vi "WHD_VEten_0.1.4.WS_BIDIR_Cal_05_03_2020 - modificado.vi"() -> ()   [LabVIEW 2015]
uses:
  <vilib>/LabVIEW Targets/FPGA/cRIO/shared/nicrio_ModuleControls/nicrio_cRIO-9234_DataRatesRing2.ctl
  <vilib>/RTwatchdog.llb/Watchdog expiration actions.ctl
  <vilib>/userdefined/High Color/nirio_resource_hc.ctl
  <vilib>/Platform/TimedLoop/XDataNode/timing_clust.ctl
  <vilib>/Platform/TimedLoop/XDataNode/nitl_modes.ctl
  <vilib>/Platform/TimedLoop/XDataNode/wakeup.ctl
  <vilib>/Analysis/5stat.llb/RMS (DBL).vi
  <vilib>/FPGAPlugInAG/cRIO-9031/niLvFpga_Open_cRIO-9031.vi
  <vilib>/Utility/error.llb/Error Cluster From Error Code.vi
  <vilib>/rvi/errors/niLvFpgaAdjustHostInterfaceError.vi
  <vilib>/FPGAPlugInAG/cRIO-9031/niLvFpga_Run_cRIO-9031.vi
  <vilib>/rvi/interface/common/niFpgaWaitOnOcc.vi
  <vilib>/Utility/file.llb/Write Delimited Spreadsheet (string).vi
  <vilib>/FPGAPlugInAG/cRIO-9031/niLvFpga_Reset_cRIO-9031.vi
  <vilib>/measure/madcrms.llb/Basic Averaged DC-RMS for 1 Chan.vi
  <vilib>/measure/maspectr.llb/FFT Spectrum (Mag-Phase) for 1 Chan.vi
  <vilib>/Utility/config.llb/Write Key (Double).vi
  <vilib>/FPGAPlugInAG/cRIO-9031/niLvFpga_Close_cRIO-9031.vi
  <vilib>/rvi/interface/nirviOpenFPGA/nirviOpenFPGA.xnode
  FPGA Bitfiles/WRDArabia_FPGATarget_FPGA8a2wsBIdirec_pdg683fU6LY.lvbitx
  <vilib>/rvi/interface/nirviReadWriteControl/nirviReadWriteControl.xnode
  <vilib>/rvi/interface/nirviMethod/nirviMethod.xnode
  <vilib>/platform/TimedLoop/XDataNode/XDataNode.xnode
  <vilib>/rvi/interface/nirviCloseFPGA/nirviCloseFPGA.xnode
  <vilib>/rvi/errors/niLvFpgaMergeErrorWithErrorCode.vi
  AURA_Wheel/Json2Labv.lvlib
  AURA_Wheel/AuraWheelAPI/AuraWheel.lvlib
  NiFpgaLv.dll
  <vilib>/FPGAPlugInAG/cRIO-9031/niLvFpga_ConfigureFifo_cRIO-9031.vi
  <vilib>/FPGAPlugInAG/cRIO-9031/niLvFpga_StartFifo_cRIO-9031.vi
  <vilib>/FPGAPlugInAG/cRIO-9031/niLvFpga_ReadFifo_cRIO-9031.vi
  <vilib>/FPGAPlugInAG/cRIO-9031/niLvFpga_StopFifo_cRIO-9031.vi
  <vilib>/measure/NI_MAPro.lvlib
  <vilib>/Analysis/NI_AALPro.lvlib
  <vilib>/Analysis/NI_AALBase.lvlib
  <vilib>/Utility/config.llb/NI_LVConfig.lvlib
  <vilib>/Platform/TimedLoop/XDataNode/XDNodeRunTimeDep.lvlib
  Library/IF2_Reader/IF2_Reader.lvlib
panel:
  out "appended array":string[][](array[string])
  out "TagData out":cluster{"TagCode":string, "FirstSeemUs":u64}[](array[cluster])
  out "error_RFID":errorcluster
  out "Power Status":bool
  out "Diagnostic data":sgl[](array[numeric])
  out "Last Train passes - RFIDs":T1
  out "I2":sgl[](array[numeric])
  out "I1":sgl[](array[numeric])
  out "A8":sgl[](array[numeric])
  out "A7":sgl[](array[numeric])
  out "A6":sgl[](array[numeric])
  out "A5":sgl[](array[numeric])
  out "A4":sgl[](array[numeric])
  out "A3":sgl[](array[numeric])
  out "A2":sgl[](array[numeric])
  out "A1":sgl[](array[numeric])
  out "Accelerometer 8":bool
  out "Accelerometer 7":bool
  out "Accelerometer 6":bool
  out "Accelerometer 5":bool
  out "Accelerometer 4":bool
  out "Accelerometer 3":bool
  out "Accelerometer 2":bool
  out "Accelerometer 1":bool
  out "Wheel detector 2":bool
  out "Wheel Detector 1":bool
  out "Last time checked":string
  out "RFID connection":bool
  out "Internet connection":bool
  out "Inicio diagnosis":timestamp
  out "RFID_status":path=path "c:/RFID/status.csv"
  in  "Diagnosis":bool
  out "T fuera rango":bool
  out "Frequency":dbl[](array[numeric])
  out "Value to compare":dbl[](array[numeric])
  in  "Developer password":string
  out "min":dbl[](array[numeric])
  out "max":dbl[](array[numeric])
  out "median":dbl[](array[numeric])
  out "mean":dbl[](array[numeric])
  in  "Accelerometer":i32=1 min=1 max=8
  out "Low cutoff freq":dbl
  out "noise_range":dbl
  out "Numeric":i32
  out "Calibration parameter":dbl
  out "Accel.detected":i32
  out "Mean\nfrequency":dbl format="%0.2f"
  out "Nº meas":i32
  out "Array":i32[](array[numeric])
  out "sorted array":i32[](array[numeric])
  out "Array 3":i32[](array[numeric])
  out "max value":i32
  out "max index(es)":i32
  out "element":i32
  out "size(s) 3":i32
  out "size(s)":i32[](array[numeric])
  out "Valid\nindex":i32[](array[numeric])
  out "Acquiring time":dbl
  out "Inicio pasada 2":timestamp
  out "calibration log":path
  out "date/time string 2":string
  out "Folder":path
  in  "Developer commad":string
  out "Save calibration":bool
  out "Pattern amplitude (g)":dbl=1.02
  out "Pattern frequency (Hz)":dbl=159.2
  out "Report":string
  out "AURA wheel test":bool
  out "LOG.txt":path
  out "Report_AURA":string
  out "error FPGA":errorcluster
  out "error AURA":errorcluster
  out "error manipulacion archivos":errorcluster
  out "Response headers":string
  out "Max RMS Ruedas":dbl[][](array[numeric])
  out "TAGs LR6":string[](array[string])
  out "TAGs HEX":string[](array[string])
  out "Parar":bool
  out "result":bool
  out "TAGs":string[](array[string])
  out "Temperatura (ºC)":dbl
  out "V (m/s)":dbl
  out "Digital?":bool=TRUE
  out "Watchdog config":T2={"reset"=FALSE, "occurrence"=FALSE, "trigger protocol"=enum."active high", "trigger line"=enum."none", "disable watchdog on VI exit"=TRUE}
  out "Tiempo de adquisicion":dbl=10.0
  out "Adquirir":bool
  out "Nº Ruedas 1":i32
  out "NºRuedas 2":i32
  out "Disco Duro Disponible (bytes)":i64
  out "Buffer Overflow":bool
  out "Buffer Underflow":bool
  out "Archivo\nvalido?":bool
  out "Número de ejes detectados":i32
  out "Ejes_convoy":i32
  out "Tiempo de paso (s)":dbl
  out "created path":path
  out "Nombre de archivo":path[](array[path])
  out "LR6 IP address":string="192.168.106.94"
  out "Port LR6":u16=2001
  out "Frecuencia de muestreo (Hz)":dbl=25600.0
  out "Escaneos de la FIFO por canal":u32=5000
  out "Tiempo extra al detector de paso (s)":dbl=1.0
  out "dt RMS":dbl=256.0
  out "Frecuencia de muestreo y módulo CRIO":T3=2 items=["51.200 kS/s (NI 9234)"=1, "25.600 kS/s (NI 9234)"=2, "17.067 kS/s (NI 9234)"=3, "12.800 kS/s (NI 9234)"=4, "10.240 kS/s (NI 9234)"=5, "8.533 kS/s (NI 9234)"=6, "7.314 kS/s (NI 9234)"=7, "6.400 kS/s (NI 9234)"=8, "5.689 kS/s (NI 9234)"=9, "5.120 kS/s (NI 9234)"=10, "4.654 kS/s (NI 9234)"=11, "4.267 kS/s (NI 9234)"=12, "3.938 kS/s (NI 9234)"=13, "3.657 kS/s (NI 9234)"=14, "3.413 kS/s (NI 9234)"=15, "3.200 kS/s (NI 9234)"=16, "3.012 kS/s (NI 9234)"=17, "2.845 kS/s (NI 9234)"=18, "2.695 kS/s (NI 9234)"=19, "2.560 kS/s (NI 9234)"=20, "2.438 kS/s (NI 9234)"=21, "2.328 kS/s (NI 9234)"=22, "2.226 kS/s (NI 9234)"=23, "2.133 kS/s (NI 9234)"=24, "2.048 kS/s (NI 9234)"=25, "1.969 kS/s (NI 9234)"=26, "1.896 kS/s (NI 9234)"=27, "1.829 kS/s (NI 9234)"=28, "1.765 kS/s (NI 9234)"=29, "1.707 kS/s (NI 9234)"=30, "1.652 kS/s (NI 9234)"=31]
  out "Puerto RFID":u16=2189
  out "IP RFID":string="192.168.106.99"
  out "Offset_rueda WS 2":fxp<+/-,24,-4>=0.004999998956918716 format="%.27g"
  out "Count(mSec)":u32=2
  out "RFID NEM on?":bool
  out "RFID LR6 on?":bool
  out "Canal cero WS1?":bool
  out "Canal cero WS2":bool
  in  "Calibration":bool
  out "Direccion 0?":bool
  out "Boton Adquirir?":bool
  out "RuedaDetectada2?":bool=TRUE
  out "RuedaDetectada1?":bool=TRUE
  out "Timeout ruedas":dbl
  out "Borrar archivos\nadquisicion con error":bool
  out "Able watchdog?":bool
  out "Reset watchdog?":bool
  out "Leer config RFID NEM":bool
  out "bytes to read":i32
  out "DeviceAddress":u8
  out "timeout ms (60000)":i32
  out "Max archivos":u32=2
  out "Bytes libre despues de borrar":u32=2
  out "Bytes min libre":u32=2
  out "Nº de acelerómetros":i32
  out "Nº inductivos":i32
  out "Offset_rueda WS 1":fxp<+/-,24,-4>=0.004999998956918716 format="%.27g"
  out "TAGs_AURAwheel":string[][](array[string])
  out "Plataformas?":bool
  out "Nº Ejes":i32[](array[numeric])
  out "Nº UTs":i32
  out "it-read-LR6":i32[](array[numeric])
  out "it-LR6":i32
  out "RFID_LR6_Error":errorcluster
  out "Series_flota":string[](array[string])
  out "Tabla_flota":string[][](array[string])
  out "Puntos medios de las ventanas":dbl[][](array[numeric])
  out "configuration file path":path=path "c:/Parametros.cfg"
  out "IP synchr":string
  out "data":cluster{"status":string}
  out "confRFID":path=path "c:/RFID/TAGS.csv"
  out "TAGS leidos":path=path "c:/RFID/TAGS.csv"
  out "Use Aura?":bool
  out "Parametros AuraWheel":string[](array[string])
  out "Parámetros acelerómetros":dbl[](array[numeric])
  out "Fin":bool
  out "Contador":i32=1
  out "Path LOG":path=path "c:/TEST"
  out "Fallo fotocelula":bool
  out "Path_Borrar":path=path "c:/Trenes"
  out "Longitud de la unidad":dbl
  out "Aviso no detección":string
  out "Time to Acquire Block (ms)":i32
  out "Distancia de acelerómetros":dbl[](array[numeric])
  out "Block Size":u32
  out "Distancias generales":dbl[](array[numeric])
  out "Reset del controlador":bool
  out "Parar la aplicación":bool
  out "date/time string":string
  out "Timeout ruedas":bool
  out "Tiempo":dbl
  out "Inicio pasada":timestamp
  out "Ultimo TEST":timestamp
  out "DC OK":string
  out "Aviso temperatura":string
  out "connection ID":refnum<k5>
  # "Date"
  # "Train"
  # "TAG1"
  # "TAG2"
  # "To check the status of the UPS please check the following LEDs physically in the system:"
  # "10. Bar graph showing the current available supply of the UPS (each bar is a 20%)"
  # "12. Red LED: alarm"
  # "13. Yellow LED: battery working mode"
  # "16. Green LED: Power In OK, mains mode"
  # "Calibration - Noise analysis"
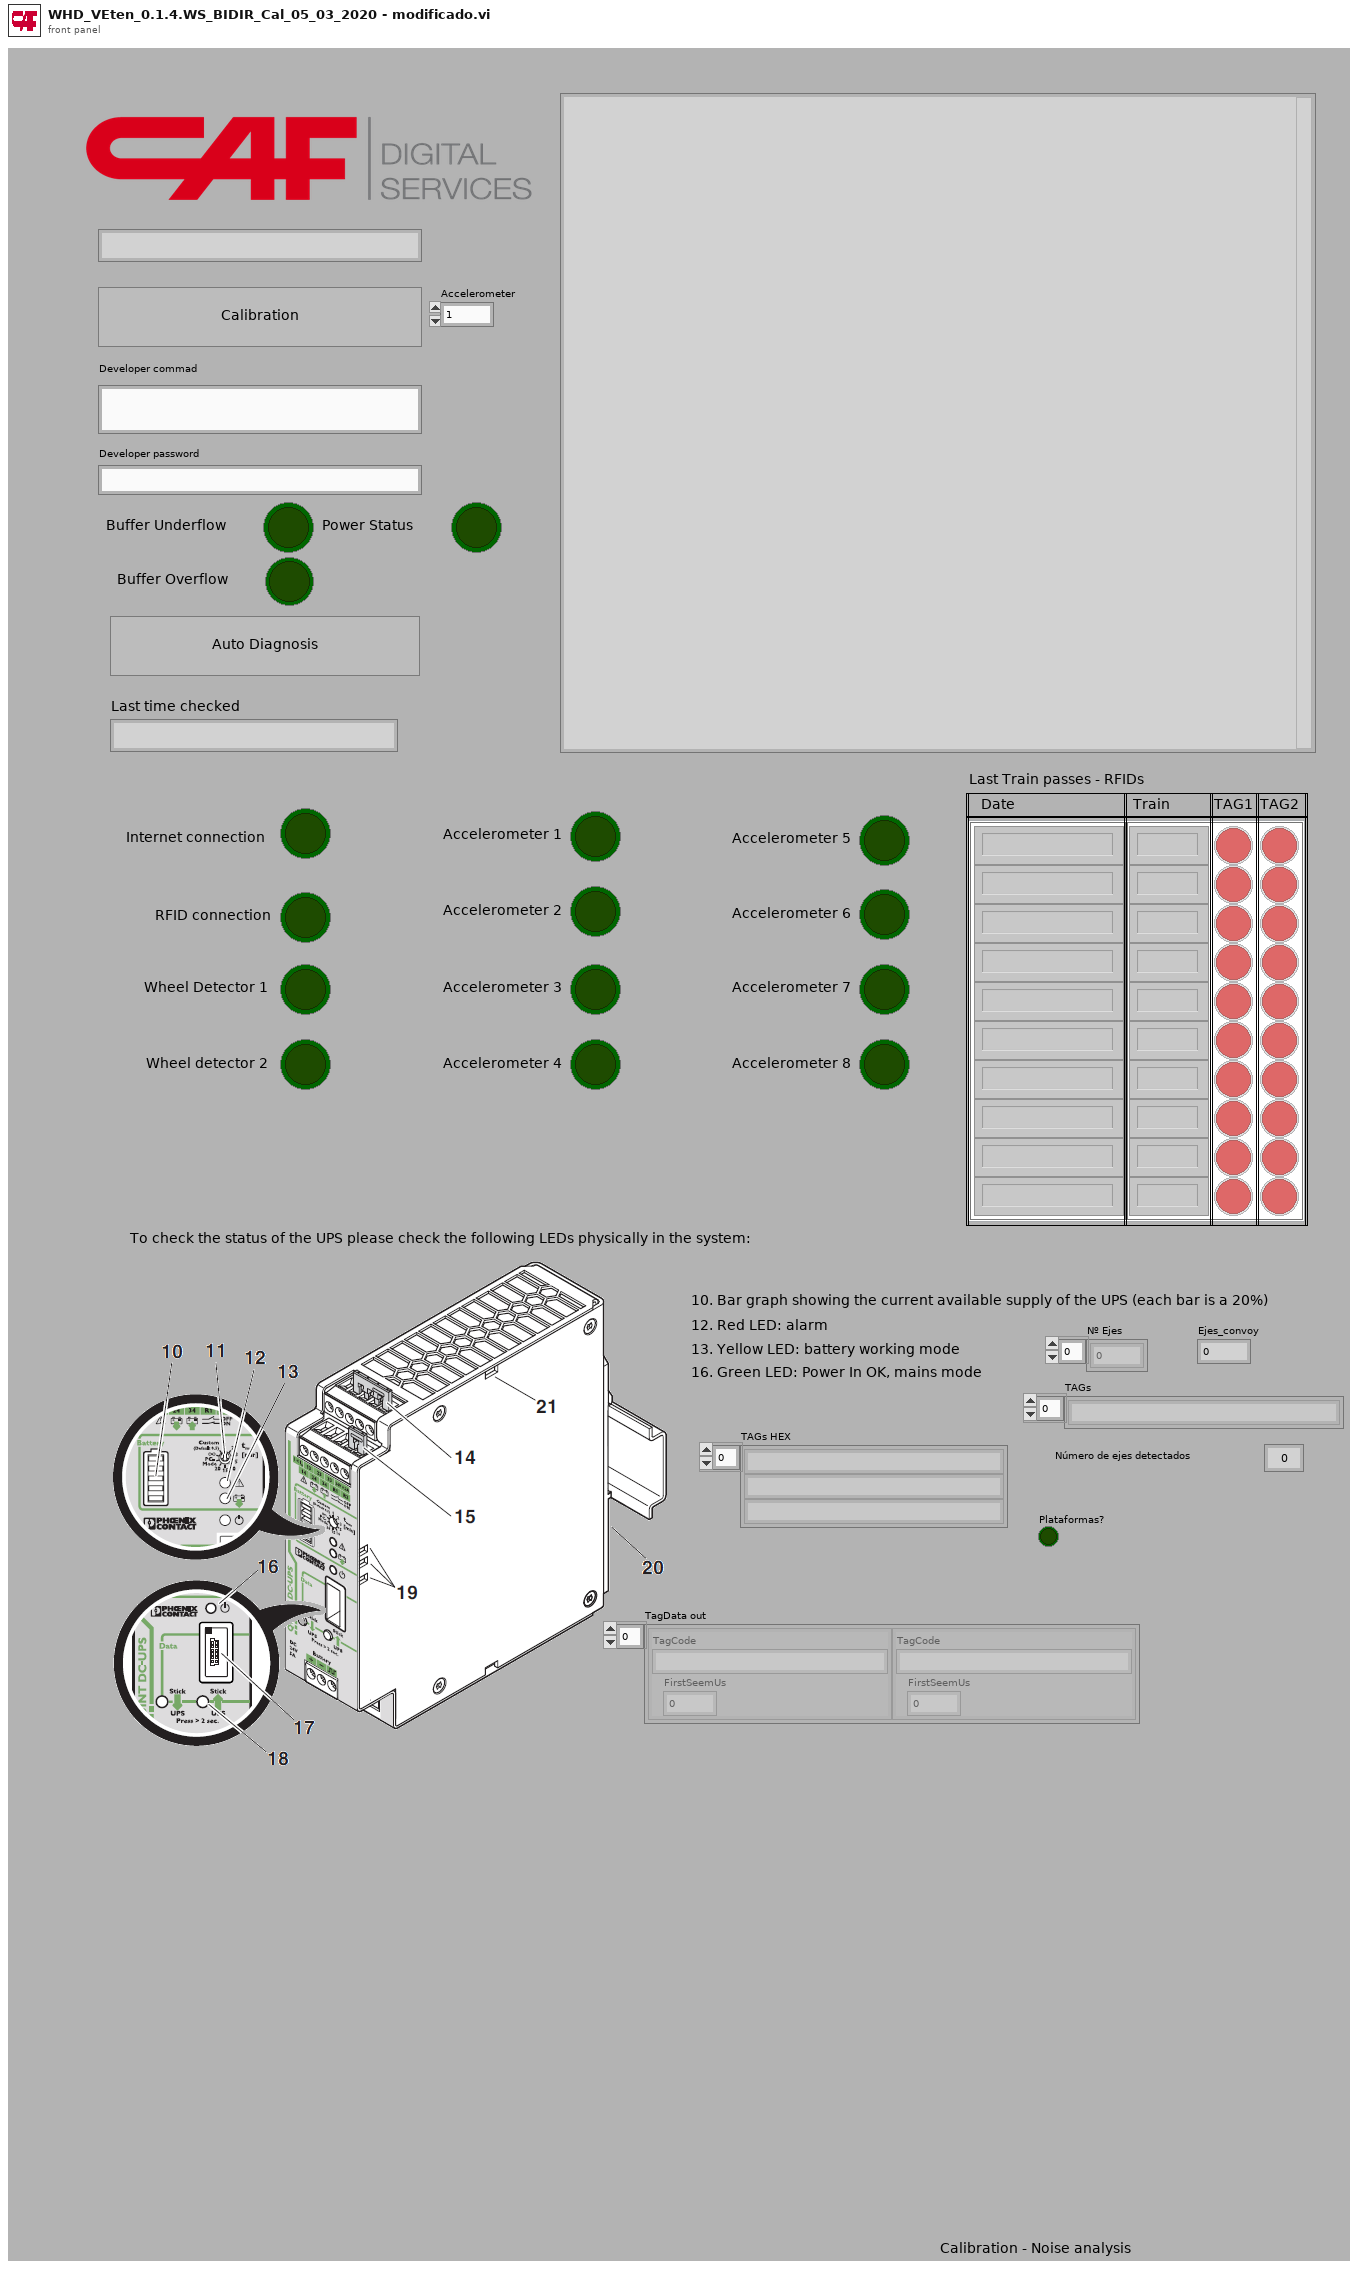
[diagram p1: front panel]
types:
  T1 = cluster{"Array 3":bool[], "Array 4":string[], "Array 6":string[], "Array 5":bool[]}
  T2 = typedef "Watchdog expiration actions.ctl" = cluster{"reset":bool, "occurrence":bool, "trigger protocol":enum16{"active high", "active low", "open collector"}, "trigger line":enum16{"none", "line 0", "line 1", "line 2", "line 3", "line 4", "line 5", "line 6", "line 7", "SMB line 0"}, "disable watchdog on VI exit":bool}
  T3 = typedef "nicrio_cRIO-9234_DataRatesRing2.ctl" = u8
  T4 = typedef "nirio_resource_hc.ctl" = tag
  T5 = enum16{"open", "replace", "create", "open or create", "replace or create", "replace or create with confirmation"}
  T6 = enum16{"big-endian, network order", "native, host order", "little-endian"}
  T7 = typedef "XDNodeRunTimeDep.lvlib/timing_clust.ctl" = cluster{"Expected End [f-1]":u64, "Actual End [f-1]":u64, "Finished Late? [f-1]":bool, "Expected End [i-1]":u64, "Actual End [i-1]":u64, "Finished Late? [i-1]":bool, "Expected Start [i]":u64, "Actual Start [i]":u64, "Expected Start [f]":u64, "Actual Start [f]":u64, "Source Name":string, "Structure Name":string, "Period":i64, "Deadline":i64, "Offset":i64, "Start":i64, "Priority":i32, "Timeout":i32, "Mode":T8, "Wakeup Reason":T9, "Error":errorcluster, "Source Type":string, "Secondary Source Type":string, "Global End Time":u64, "Global Start Time":u64, "Frame Duration":u64, "Iteration Duration":u64, "Assigned CPU":i32, "I/O Scan Engine Mode":u32}
  T8 = typedef "XDNodeRunTimeDep.lvlib/nitl_modes.ctl" = enum32{"No Change", "Process missed periods, maintain original phase", "Discard missed periods, maintain original phase", "Process missed periods, ignore original phase", "Discard missed periods, ignore original phase"}
  T9 = typedef "XDNodeRunTimeDep.lvlib/wakeup.ctl" = enum32{"Normal", "Aborted", "Asynchronous wakeup", "Timing source error", "Timed loop error", "Timeout"}
  T10 = cluster{"error IO":errorcluster, bool[], u32[], string[], dbl[]}
  T11 = cluster{"error out":errorcluster, dbl[], "Normalized Tags":string[], "Direccion 0?":bool}
  T12 = cluster{"g_ts":dbl, "p_sp":dbl, "p_tp":dbl, "p_tg":cluster{"tg_n":dbl, "tg_t":string}[], "p_ax":cluster{"ax_n":dbl, "ax_sp":dbl, "ax_wh":cluster{"wh_p":dbl, "wh_a1":dbl, "wh_a2":dbl, "wh_a3":dbl, "wh_a4":dbl}[]}[]}
  T13 = typedef "NI_LVConfig.lvlib/Config Data RefNum.ctl" = refnum<k1>
  T14 = cluster{"IP":string, "Port":u16, "ReaderConfigFile":path, "ROspecConfigFile":path}
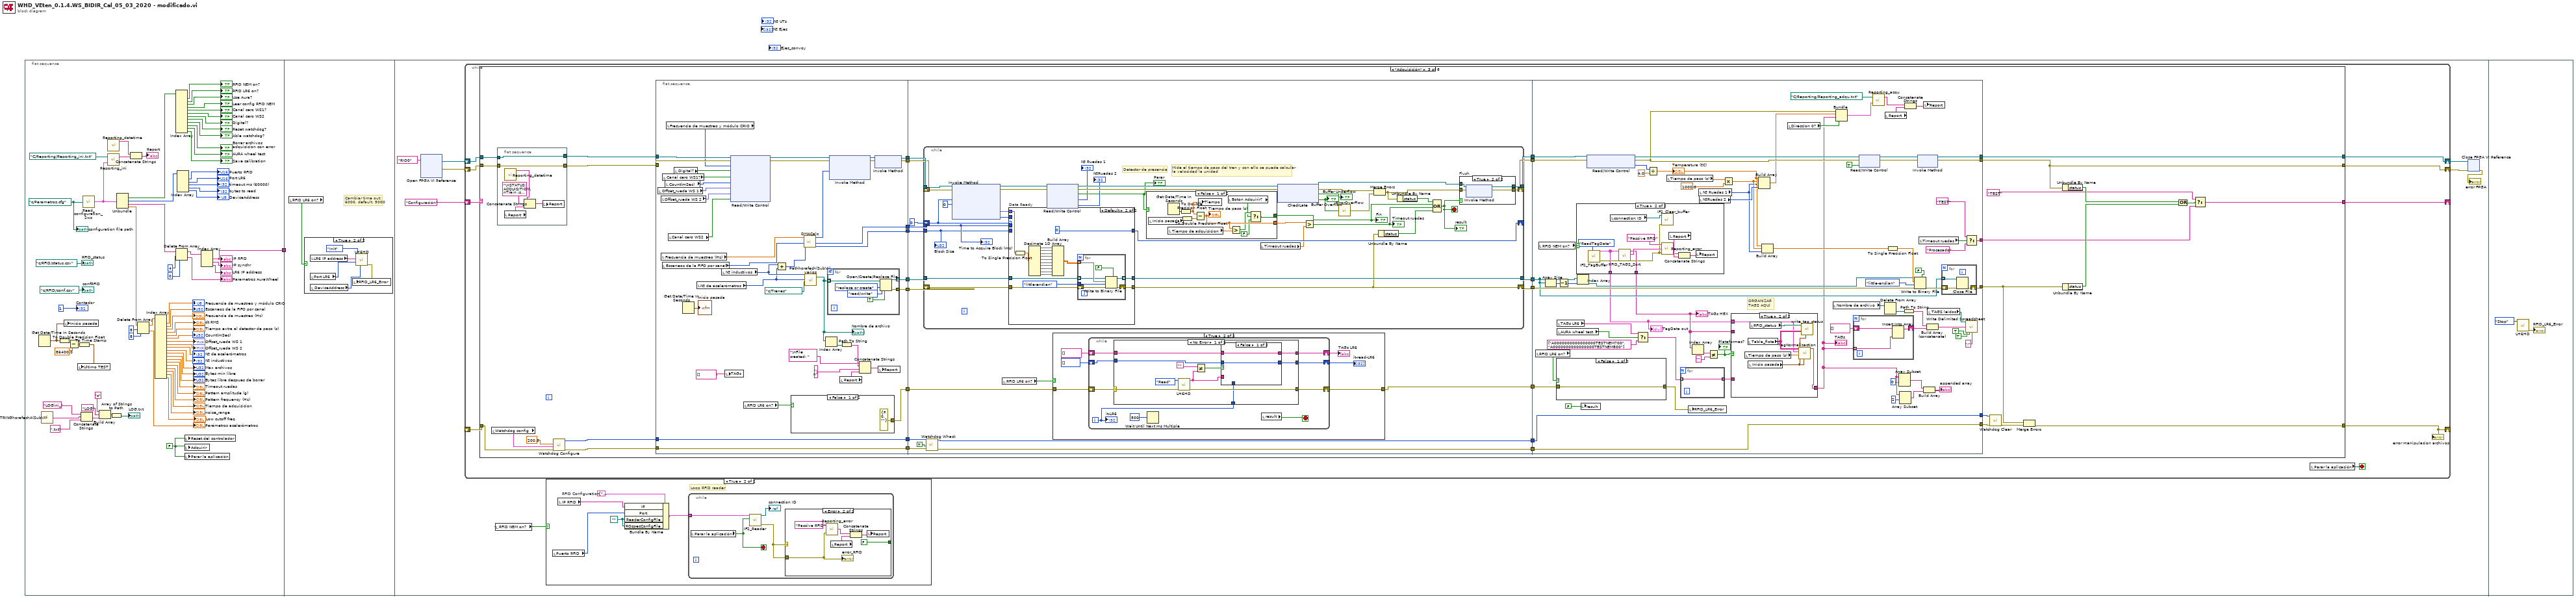
[diagram p0: block diagram]
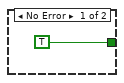
[diagram p4: hidden frame]
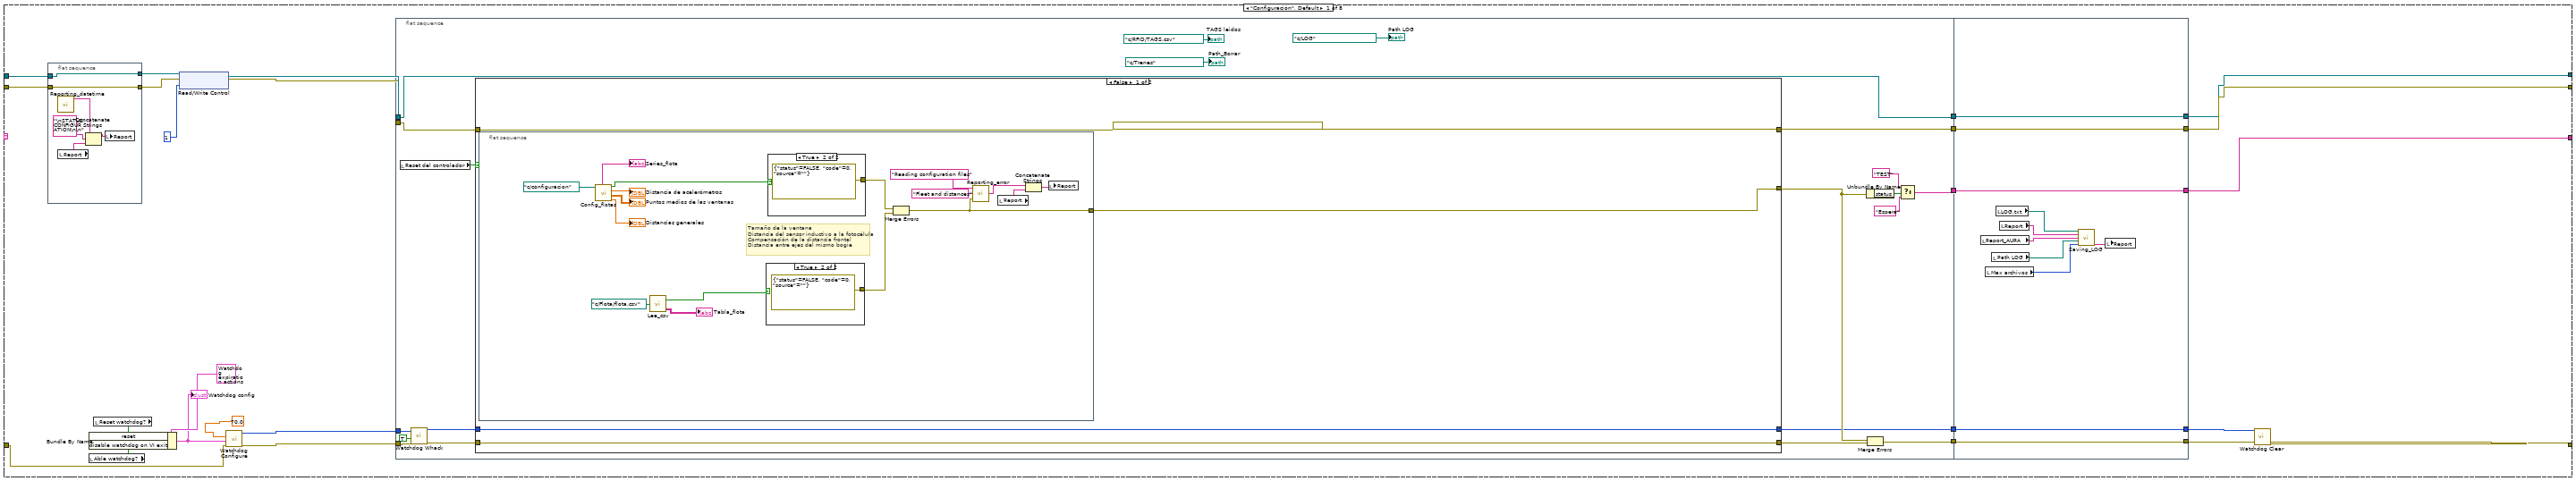
[diagram p5: hidden frame]
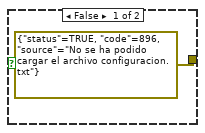
[diagram p6: hidden frame]
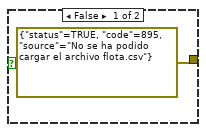
[diagram p7: hidden frame]
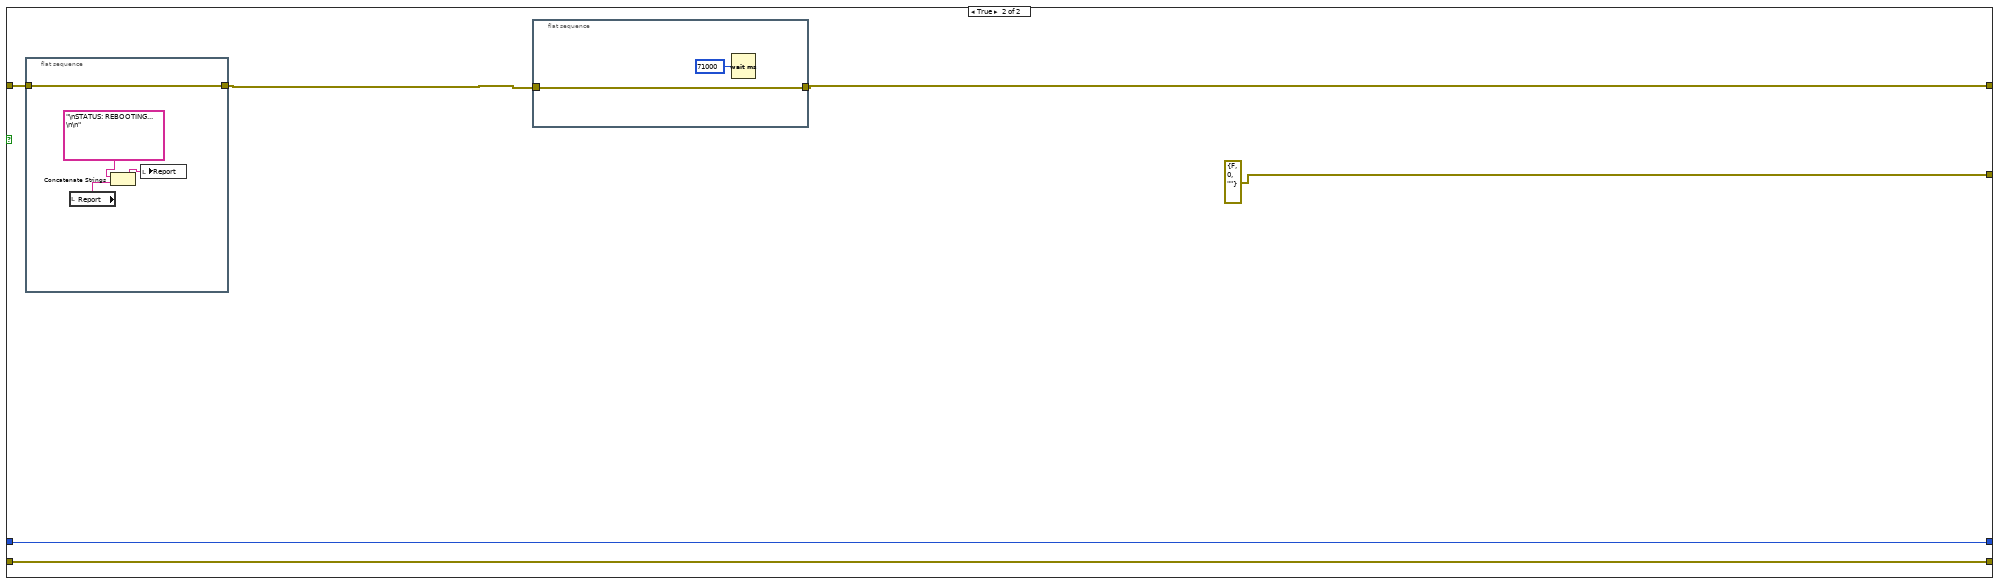
[diagram p8: hidden frame]
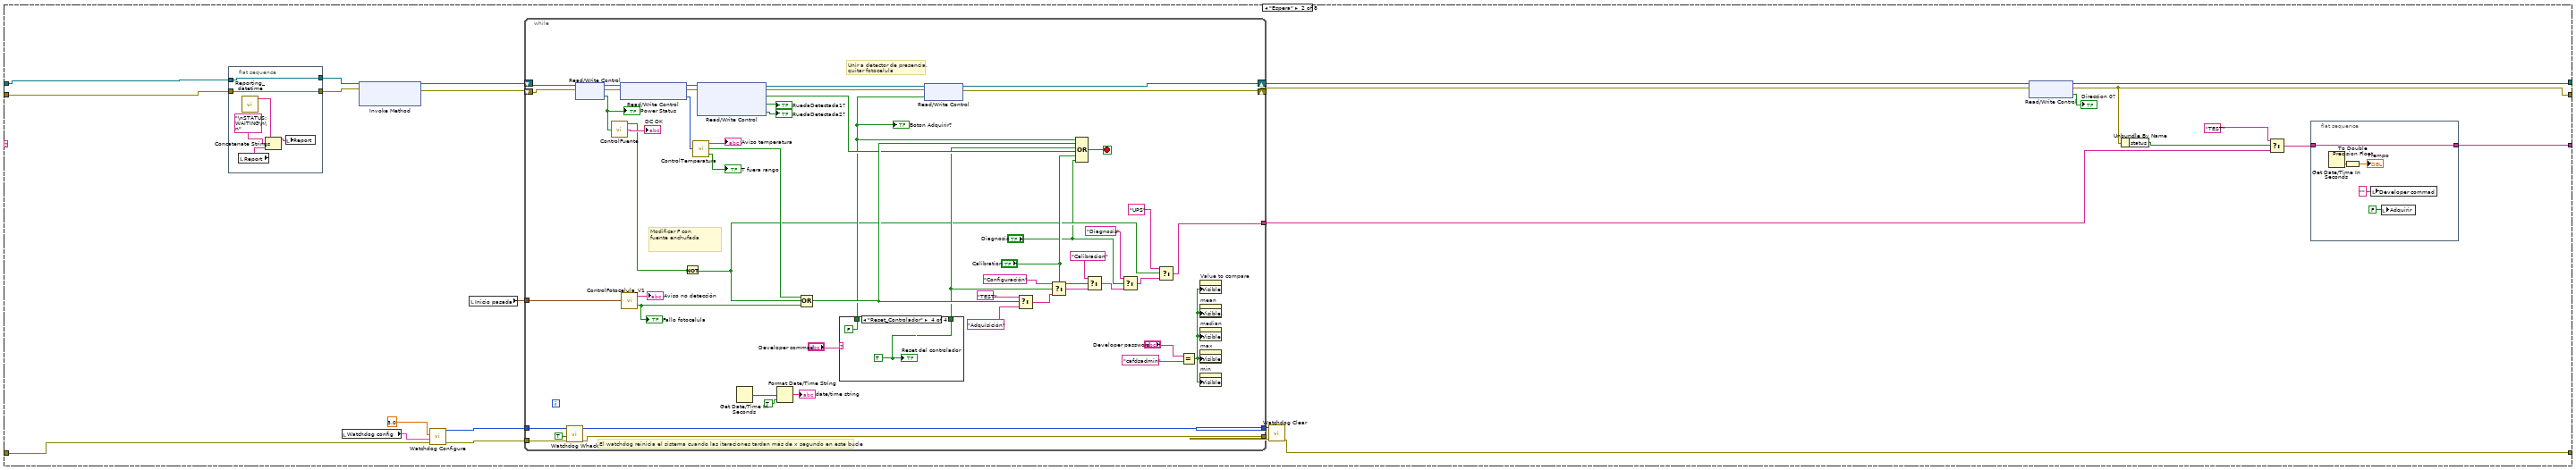
[diagram p9: hidden frame]
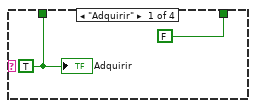
[diagram p10: hidden frame]
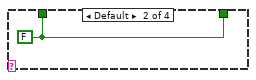
[diagram p11: hidden frame]
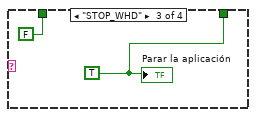
[diagram p12: hidden frame]
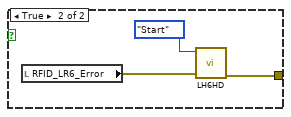
[diagram p13: hidden frame]
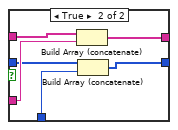
[diagram p15: hidden frame]
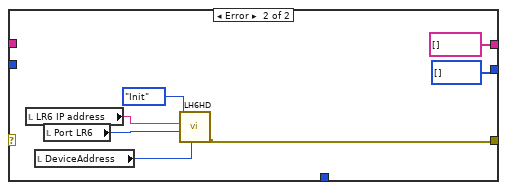
[diagram p16: hidden frame]
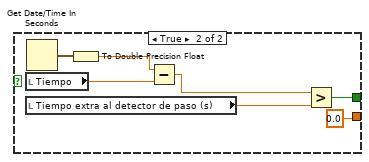
[diagram p17: hidden frame]
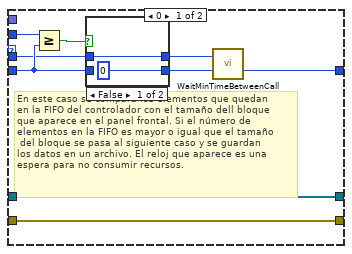
[diagram p18: hidden frame]
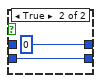
[diagram p19: hidden frame]
diagram:
  n1 = flat-sequence {
    tunnel: [w5] -> w1
    tunnel: w1 -> [_]
    frame #0 {
      w6 = FALSE ("Reset del controlador")
      w67 = path "c:/Parametros.cfg" ("configuration file path")
      n2 = Get Date/Time In Seconds() -> (seconds since 1Jan1904=w72:timestamp)
      n3 = call "STRINGhorafechA(SubVI).vi"() -> ("STRINGhora_fecha"=w17:string)
      n4 = To Double Precision Float(number=w72) -> (double precision float=w74:dbl)
      n5 = local write "Inicio pasada"(w72) -> ()
      n6 = Subtract(x=w74, y=86400.0) -> (x-y=w73:dbl)
      n7 = To Time Stamp(1:w73) -> (0:w71:timestamp)
      n8 = local write "Ultimo TEST"(w71) -> ()
      n9 = Concatenate Strings("LOGini_" ("string"), w17, ".txt" ("string")) -> (w19:string)
      n10 = call "Read_configuration_2ws.vi"("configuration file path"=w67) -> ("output cluster"=w23:T10)
      n11 = Build Array("c", "LOG" ("element"), w19) -> (w16:string[])
      n12 = call "Reporting_ini.vi"("Configuration cluster"=w23, "address repoting"=path "C:/Reporting/Reporting_ini.txt" ("file (use dialog)")) -> ("Reporting"=w22:string)  [unwired: 1 in]
      n13 = call "Reporting_datetime.vi"() -> ("String"=w20:string)  [unwired: 11 in]
      n14 = Array of Strings to Path(0:w16) -> (2:→"LOG.txt":path)  [unwired: 1 out]
      n15 = Unbundle(w23) -> (w70:bool[], w69:u32[], w62:string[], w66:dbl[])  [unwired: 1 out]
      n16 = Concatenate Strings(w20, w22) -> (→"Report":string)
      n17 = Delete From Array(array=w66, length=8, index=8) -> (deleted portion=→"Parámetros acelerómetros":dbl[], array with subset deleted=w65:dbl[])
      n18 = Index Array(array=w65) -> (element #1=→"Frecuencia de muestreo y módulo CRIO":dbl, element #2=→"Escaneos de la FIFO por canal":dbl, element #3=→"Frecuencia de muestreo (Hz)":dbl, element #4=→"dt RMS":dbl, element #5=→"Tiempo extra al detector de paso (s)":dbl, element #6=→"Count(mSec)":dbl, element #7=→"Offset_rueda WS 1":dbl, element #8=→"Offset_rueda WS 2":dbl, element #9=→"Nº de acelerómetros":dbl, element #10=→"Nº inductivos":dbl, element #11=→"Max archivos":dbl, element #12=→"Bytes min libre":dbl, element #13=→"Bytes libre despues de borrar":dbl, element #14=→"Timeout ruedas":dbl, element #15=→"Pattern amplitude (g)":dbl, element #16=→"Pattern frequency (Hz)":dbl, element #17=→"Tiempo de adquisicion":dbl, element #18=→"noise_range":dbl, element #19=→"Low cutoff freq":dbl)  [unwired: 19 in]
      n19 = Index Array(array=w70) -> (element #1=→"RFID NEM on?":bool, element #2=→"RFID LR6 on?":bool, element #3=→"Use Aura?":bool, element #4=→"Leer config RFID NEM":bool, element #5=→"Canal cero WS1?":bool, element #6=→"Canal cero WS2":bool, element #7=→"Digital?":bool, element #8=→"Reset watchdog?":bool, element #9=→"Able watchdog?":bool, element #10=→"Borrar archivos\nadquisicion con error":bool, element #11=→"AURA wheel test":bool, element #12=→"Save calibration":bool)  [unwired: 12 in]
      n20 = Delete From Array(array=w62, length=4, index=0) -> (deleted portion=→"Parametros AuraWheel":string[], array with subset deleted=w61:string[])
      n21 = Index Array(array=w69) -> (element #1=→"Puerto RFID":u32, element #2=→"Port LR6":u32, element #3=→"timeout ms (60000)":u32, element #4=→"bytes to read":u32, element #5=→"DeviceAddress":u32)  [unwired: 5 in]
      n22 = local write "Reset del controlador"(w6) -> ()
      n23 = local write "Adquirir"(w6) -> ()
      n24 = local write "Parar la aplicación"(w6) -> ()
      n25 = Index Array(array=w61) -> (element #1=w5:string, element #2=→"IP synchr":string, element #3=→"LR6 IP address":string)  [unwired: 3 in]
      "IP RFID" <- w5
      "Contador" <- 1
      "confRFID" <- path "c:/RFID/conf.csv" ("file path (use dialog)")
      "configuration file path" <- w67
      "RFID_status" <- path "c:/RFID/status.csv" ("file path (use dialog)")
    }
    frame #1 {
      # "Cambiar time out:\n6000, default, 5000"
      n26 = local read "RFID LR6 on?"() -> (w76:bool)
      n27 = case shown="True" w76 {
        frame False {
        }
        frame True {
          n28 = local read "LR6 IP address"() -> (w77:string)
          n29 = local read "Port LR6"() -> (w78:u16)
          n30 = local read "DeviceAddress"() -> (w79:u8)
          n31 = call "LH6HD.vi"("DeviceAddress"=w79, "Reader Port"=w78, "IP Address"=w77, "Action"=enum16{"Init", "Start", "Read", "Stop", "Exit"}."Init") -> ("error out"=w81:errorcluster)  [unwired: 6 in, 1 out]
          n32 = local write "RFID_LR6_Error"(w81) -> ()
        }
      }
    }
    frame #2 {
      n33 = xnode "Open FPGA VI Reference"("resource name"=T4 "RIO0") -> ("FPGA VI Reference Out"=w89:refnum<k20>, "error out"=w88:errorcluster)  [unwired: 1 in]
      n34 = while {
        shift-right: [w107] -> _
        shift-left: "Configuración" -> [w114]
        shift-right: [w106] -> w85
        shift-left: w89 -> [w113]
        shift-right: [w108] -> w84
        shift-left: w88 -> [w112]
        shift-right: [w111] -> _
        shift-left: _ -> [w110]
        stop <- w109 stop-if-true
        n35 = case shown="\"Adquisición\"" w114 {
          tunnel: [w129 w232 w328 w682 w931 "Espera" "Espera" ("t") "Espera" ("t")] -> w107
          tunnel: [w139 w221 w342 w671 w930 w999 w1795 w1818] -> w106
          tunnel: [w140 w220 w343 w669 w929 w997 w1794 w1827] -> w108
          tunnel: w113 -> [w123 w219 w314 w672 w930 w1009 w1796 w1836]
          tunnel: w112 -> [w122 w218 w313 w670 w922 w1008 w1791 w1838]
          tunnel: [w136 w226 w340 w667 w921 w998 w1792 w1819] -> w111
          tunnel: w110 -> [w128 w231 w324 w681 w918 w998 w1792 w1819]
          frame "Configuración", Default {
            n36 = flat-sequence {
              tunnel: w123 -> [w146]
              tunnel: w122 -> [w145]
              tunnel: [w146] -> w121
              tunnel: [w145] -> w120
              frame #0 {
                n37 = call "Reporting_datetime.vi"() -> ("String"=w141:string)  [unwired: 11 in]
                n38 = local read "Report"() -> (w142:string)
                n39 = Concatenate Strings(w141, "\nSTATUS: CONFIGURATION\n\n", w142) -> (w144:string)
                n40 = local write "Report"(w144) -> ()
              }
            }
            n41 = local read "Able watchdog?"() -> (w133:bool)
            n42 = local read "Reset watchdog?"() -> (w134:bool)
            n43 = Bundle By Name(cluster=T2 {"reset"=FALSE, "occurrence"=FALSE, "trigger protocol"=enum."active high", "trigger line"=enum."none", "disable watchdog on VI exit"=TRUE} ("expiration actions"), "reset"=w134, "disable watchdog on VI exit"=w133) -> (w127:T2)
            "Watchdog config" <- w127
            n44 = xnode "Read/Write Control"("FPGA VI Reference In"=w121, "error in"=w120, "Cycles to Filter"=u16 1) -> ("FPGA VI Reference Out"=w132:refnum<k20>, "error out"=w131:errorcluster)
            n45 = call <vilib>:"Watchdog Configure.vi"("error in (no error)"=w128, "expiration actions"=w127, "timeout (1 sec)"=70.0) -> ("error out"=w124:errorcluster, "watchdogID"=w125:u64)  [unwired: 1 in, 2 out]
            n46 = flat-sequence {
              tunnel: w132 -> [w158]
              tunnel: w131 -> [w155]
              tunnel: w125 -> [w148]
              tunnel: w124 -> [w147]
              tunnel: [w157] -> w119
              tunnel: [w165] -> w118
              tunnel: [w158] -> w117
              tunnel: [w160] -> w116
              tunnel: [w152] -> w115
              tunnel: [w210] -> w138
              tunnel: [w211] -> w137
              tunnel: [w212] -> w139
              tunnel: [w213] -> w129
              tunnel: [w214] -> w140
              tunnel: w119 -> [w214]
              tunnel: w118 -> [w213]
              tunnel: w117 -> [w212]
              tunnel: w116 -> [w211]
              tunnel: w115 -> [w210]
              frame #0 {
                n47 = local read "Reset del controlador"() -> (w154:bool)
                n48 = call <vilib>:"Watchdog Whack.vi"("error in (no error)"=w147, "reset watchdog after expire? (F)"=TRUE, "watchdogID in"=w148) -> ("error out"=w150:errorcluster, "watchdogID out"=w151:u64)  [unwired: 2 in, 1 out]
                n49 = case shown="False" w154 {
                  tunnel: w155 -> [w170 w193]
                  tunnel: [w170 w196] -> w157
                  tunnel: [w167 errorcluster {"status"=FALSE, "code"=0, "source"=""} ("error IO")] -> w156
                  tunnel: [w169 w195] -> w152
                  tunnel: w151 -> [w169 w195]
                  tunnel: w150 -> [w168 w194]
                  tunnel: [w168 w194] -> w149
                  frame False {
                    n50 = flat-sequence {
                      tunnel: [w171] -> w167
                      frame #0 {
                        # "Tamaño de la ventana\nDistancia del sensor inductivo a la fotocélula\nCompensación de la distancia frontal\nDistancia entre ejes del mismo bogie"
                        n51 = call "Config_flotas.vi"("file path (dialog if empty)"=path "c:/configuracion") -> ("Distancias generales"=→"Distancias generales":dbl[], "Puntos medios de las ventanas"=→"Puntos medios de las ventanas":dbl[][], "Distancia de acelerómetros"=→"Distancia de acelerómetros":dbl[], "Distacias y medidas de dispositivos"=w184:bool, "Series_flota"=→"Series_flota":string[])  [unwired: 3 in]
                        n52 = call "Lee_csv.vi"("Path"=path "c:/Flota/flota.csv") -> ("Tabla_flota"=→"Tabla_flota":string[][], "Lectura_OK?"=w181:bool)
                        n53 = case shown="True" w181 {
                          tunnel: [errorcluster {"status"=TRUE, "code"=895, "source"="No se ha podido cargar el archivo flota.csv"} ("error out") errorcluster {"status"=FALSE, "code"=0, "source"=""} ("error out")] -> w185
                          frame False {
                          }
                          frame True {
                          }
                        }
                        n54 = case shown="True" w184 {
                          tunnel: [errorcluster {"status"=TRUE, "code"=896, "source"="No se ha podido cargar el archivo configuracion.txt"} ("error out") errorcluster {"status"=FALSE, "code"=0, "source"=""} ("error out")] -> w186
                          frame False {
                          }
                          frame True {
                          }
                        }
                        n55 = Merge Errors(w186, w185) -> (w171:errorcluster)
                        n56 = call "Reporting_error.vi"("error out 2"=w171, "Concept explanation"="Fleet and distances", "Concept"="Reading configuration files") -> ("Reporting"=w173:string)
                        n57 = local read "Report"() -> (w172:string)
                        n58 = Concatenate Strings(w173, w172) -> (w174:string)
                        n59 = local write "Report"(w174) -> ()
                      }
                    }
                  }
                  frame True {
                    n60 = flat-sequence {
                      tunnel: w193 -> [w201]
                      tunnel: [w201] -> w192
                      frame #0 {
                        n61 = local read "Report"() -> (w200:string)
                        n62 = Concatenate Strings("\nSTATUS: REBOOTING...\n\n", w200) -> (w198:string)
                        n63 = local write "Report"(w198) -> ()
                      }
                    }
                    n64 = flat-sequence {
                      tunnel: [w203] -> w196
                      tunnel: w192 -> [w203]
                      frame #0 {
                        n65 = Wait (ms)(milliseconds to wait=u32 71000) -> ()  [unwired: 1 out]
                      }
                    }
                  }
                }
                n66 = Unbundle By Name(w156) -> ("status"=w166:bool)
                n67 = Merge Errors(w156, w149) -> (w160:errorcluster)
                n68 = Select(t="TEST", s=w166, f="Espera") -> (s? t:f=w165:string)
                "Path_Borrar" <- path "c:/Trenes" ("file path (use dialog)")
                "Path LOG" <- path "c:/LOG" ("file path (use dialog)")
                "TAGS leidos" <- path "c:/RFID/TAGS.csv" ("file path (use dialog)")
              }
              frame #1 {
                n69 = local read "Report_AURA"() -> (w207:string)
                n70 = local read "Max archivos"() -> (w208:u32)
                n71 = local read "Path LOG"() -> (w209:path)
                n72 = local read "LOG.txt"() -> (w204:path)
                n73 = local read "Report"() -> (w206:string)
                n74 = call "Saving_LOG.vi"("Path"=w204, "Report"=w206, "Report AURA"=w207, "Path Carpeta"=w209, "Nº Archivos Max"=w208) -> ("Report"=w205:string)  [unwired: 9 in, 1 out]
                n75 = local write "Report"(w205) -> ()
              }
            }
            n76 = call <vilib>:"Watchdog Clear.vi"("error in (no error)"=w137, "watchdogID in"=w138) -> ("error out"=w136:errorcluster)  [unwired: 5 in]
          }
          frame "Espera" {
            n77 = flat-sequence {
              tunnel: w219 -> [w245]
              tunnel: w218 -> [w244]
              tunnel: [w245] -> w217
              tunnel: [w244] -> w216
              frame #0 {
                n78 = local read "Report"() -> (w241:string)
                n79 = call "Reporting_datetime.vi"() -> ("String"=w240:string)  [unwired: 11 in]
                n80 = Concatenate Strings(w240, "\nSTATUS: WAITING\n\n", w241) -> (w243:string)
                n81 = local write "Report"(w243) -> ()
              }
            }
            n82 = local read "Watchdog config"() -> (w225:T2)
            n83 = xnode "Invoke Method"("FPGA VI Reference In"=w217, "error in"=w216) -> ("FPGA VI Reference Out"=w235:refnum<k20>, "error out"=w234:errorcluster)  [unwired: 1 in]
            n84 = call <vilib>:"Watchdog Configure.vi"("error in (no error)"=w231, "expiration actions"=w225, "timeout (1 sec)"=3.0) -> ("error out"=w230:errorcluster, "watchdogID"=w229:u64)  [unwired: 1 in, 2 out]
            n85 = local read "Inicio pasada"() -> (w239:timestamp)
            n86 = while {
              tunnel: [w261] -> w238
              shift-right: [w276] -> w222
              shift-left: w235 -> [w284]
              shift-right: [w275] -> w215
              shift-left: w234 -> [w283]
              tunnel: w239 -> [w287]
              tunnel: w230 -> [w273]
              tunnel: w229 -> [w274]
              tunnel: [w272] -> w228
              tunnel: [w271] -> w227
              stop <- w266 stop-if-true
              # "Modificar F con\nfuente enchufada"
              # "Unir a detector de presencia,\nquitar fotocelula"
              # "El watchdog reinicia el sistema cuando las iteraciones tardan más de x segundo en este bucle"
              n87 = call <vilib>:"Watchdog Whack.vi"("error in (no error)"=w273, "reset watchdog after expire? (F)"=TRUE, "watchdogID in"=w274) -> ("error out"=w271:errorcluster, "watchdogID out"=w272:u64)  [unwired: 2 in, 1 out]
              n88 = xnode "Read/Write Control"("FPGA VI Reference In"=w284, "error in"=w283) -> ("FPGA VI Reference Out"=w296:refnum<k20>, "error out"=w295:errorcluster, "DC OK"=w251:bool)
              "Power Status" <- w251
              n89 = call "ControlFuente.vi"("DC OK 3"=w251) -> ("DC OK 2"=w262:bool, "DC OK"=→"DC OK":string)  [unwired: 1 out]
              n90 = xnode "Read/Write Control"("FPGA VI Reference In"=w296, "error in"=w295) -> ("FPGA VI Reference Out"=w291:refnum<k20>, "error out"=w290:errorcluster, "Chassis Temperature"=w298:i16)
              n91 = call "ControlFotocelula_V1.vi"("Tiempo de entrada a espera"=w287) -> ("Aviso no detección"=→"Aviso no detección":string, "Boolean"=w288:bool)
              "Fallo fotocelula" <- w288
              n92 = Not(x=w262) -> (.not. x?=w260:bool)
              n93 = call "ControlTemperatura.vi"("Chassis Temperature"=w298) -> ("Aviso temperatura"=→"Aviso temperatura":string, "Boolean"=w292:bool, "T fuera rango"=→"T fuera rango":bool)
              n94 = xnode "Read/Write Control"("FPGA VI Reference In"=w291, "error in"=w290) -> ("FPGA VI Reference Out"=w286:refnum<k20>, "error out"=w285:errorcluster, "Detector de presencia"=w279:bool, "RuedaDetectada1?"=→"RuedaDetectada1?":bool, "RuedaDetectada2?"=→"RuedaDetectada2?":bool)
              n95 = Get Date/Time In Seconds() -> (seconds since 1Jan1904=w281:timestamp)
              n96 = Format Date/Time String(seconds (now)=w281, UTC format=TRUE) -> (date/time string=→"date/time string":string)  [unwired: 1 in]
              n97 = Compound Arithmetic op=OR(w292, w260, w288) -> (w289:bool)
              n98 = case shown="\"Reset_Controlador\"" "Developer commad" {
                tunnel: [w305 w306 FALSE ("Adquirir") FALSE ("Adquirir")] -> w265
                tunnel: [FALSE ("Adquirir") w306 w307 w309] -> w264
                frame "Adquirir" {
                  w305 = TRUE ("Adquirir")
                  "Adquirir" <- w305
                }
                frame Default {
                  w306 = FALSE ("Adquirir")
                }
                frame "STOP_WHD" {
                  w307 = TRUE ("Adquirir")
                  "Parar la aplicación" <- w307
                }
                frame "Reset_Controlador" {
                  w309 = TRUE ("Adquirir")
                  "Reset del controlador" <- w309
                }
              }
              "Boton Adquirir?" <- w265
              n99 = xnode "Read/Write Control"("FPGA VI Reference In"=w286, "error in"=w285, "Fotocélula"=w265) -> ("FPGA VI Reference Out"=w276:refnum<k20>, "error out"=w275:errorcluster)
              n100 = Select(t="TEST", s=w289, f="Adquisición") -> (s? t:f=w300:string)
              n101 = Select(t="Configuración", s=w264, f=w300) -> (s? t:f=w269:string)
              n102 = Compound Arithmetic op=OR(w265, w289, w264, w279, "Calibration", "Diagnosis") -> (w266:bool)
              n103 = Select(t="Calibracion", s="Calibration", f=w269) -> (s? t:f=w255:string)
              n104 = Select(t="Diagnosis", s="Diagnosis", f=w255) -> (s? t:f=w253:string)
              n105 = Select(t="UPS", s=w260, f=w253) -> (s? t:f=w261:string)
              n106 = Equal?(x="Developer password", y="cafdsadmin") -> (x = y?=w257:bool)
              n107 = property on="Value to compare" class="Arr (strict)"("Visible"=w257) -> ()  [unwired: 2 in, 2 out]
              n108 = property on="mean" class="Arr (strict)"("Visible"=w257) -> ()  [unwired: 2 in, 2 out]
              n109 = property on="median" class="Arr (strict)"("Visible"=w257) -> ()  [unwired: 2 in, 2 out]
              n110 = property on="max" class="Arr (strict)"("Visible"=w257) -> ()  [unwired: 2 in, 2 out]
              n111 = property on="min" class="Arr (strict)"("Visible"=w257) -> ()  [unwired: 2 in, 2 out]
            }
            n112 = call <vilib>:"Watchdog Clear.vi"("error in (no error)"=w227, "watchdogID in"=w228) -> ("error out"=w226:errorcluster)  [unwired: 5 in]
            n113 = xnode "Read/Write Control"("FPGA VI Reference In"=w222, "error in"=w215) -> ("FPGA VI Reference Out"=w221:refnum<k20>, "error out"=w220:errorcluster, "Direccion 0?"=→"Direccion 0?":bool)
            n114 = Unbundle By Name(w220) -> ("status"=w237:bool)
            n115 = Select(t="TEST", s=w237, f=w238) -> (s? t:f=w233:string)
            n116 = flat-sequence {
              tunnel: [w249] -> w232
              tunnel: w233 -> [w249]
              frame #0 {
                n117 = Get Date/Time In Seconds() -> (seconds since 1Jan1904=w250:timestamp)
                n118 = To Double Precision Float(number=w250) -> (double precision float=→"Tiempo":dbl)
                n119 = local write "Developer commad"("" ("Developer commad")) -> ()
                n120 = local write "Adquirir"(FALSE ("Adquirir")) -> ()
              }
            }
          }
          frame "Adquisición" {
            n121 = local read "Watchdog config"() -> (w325:T2)
            n122 = flat-sequence {
              tunnel: w314 -> [w354]
              tunnel: w313 -> [w353]
              tunnel: [w354] -> w312
              tunnel: [w353] -> w311
              frame #0 {
                n123 = local read "Report"() -> (w350:string)
                n124 = call "Reporting_datetime.vi"() -> ("String"=w349:string)  [unwired: 11 in]
                n125 = Concatenate Strings(w349, "\nSTATUS: ACQUISITION\nTrain is passing\n\n", w350) -> (w352:string)
                n126 = local write "Report"(w352) -> ()
              }
            }
            n127 = call <vilib>:"Watchdog Configure.vi"("error in (no error)"=w324, "expiration actions"=w325, "timeout (1 sec)"=200.0) -> ("error out"=w322:errorcluster, "watchdogID"=w323:u64)  [unwired: 1 in, 2 out]
            n128 = flat-sequence {
              tunnel: w311 -> [w389]
              tunnel: w312 -> [w390]
              tunnel: [w388] -> w339
              tunnel: [w387] -> w338
              tunnel: [w386] -> w337
              tunnel: [w385] -> w336
              tunnel: [w384] -> w335
              tunnel: [w383] -> w334
              tunnel: [w373] -> w327
              tunnel: w323 -> [w372]
              tunnel: w322 -> [w371]
              tunnel: [w372] -> w321
              tunnel: [w371] -> w320
              tunnel: [w405] -> w348
              tunnel: [w422] -> w347
              tunnel: [w421] -> w346
              tunnel: [w420] -> w345
              tunnel: [w413] -> w344
              tunnel: w339 -> [w419]
              tunnel: w338 -> [w418]
              tunnel: w337 -> [w417]
              tunnel: w336 -> [w416]
              tunnel: w335 -> [w415]
              tunnel: w334 -> [w414]
              tunnel: w327 -> [w411]
              tunnel: [w410] -> w326
              tunnel: w321 -> [w409]
              tunnel: w320 -> [w408]
              tunnel: [w406] -> w319
              tunnel: w348 -> [w591]
              tunnel: w347 -> [w588]
              tunnel: w346 -> [w587]
              tunnel: w345 -> [w603]
              tunnel: [w625] -> w331
              tunnel: w344 -> [w627]
              tunnel: [w618] -> w341
              tunnel: [w619] -> w343
              tunnel: [w620] -> w342
              tunnel: w326 -> [w599]
              tunnel: w319 -> [w592]
              tunnel: [w592] -> w317
              tunnel: [w591] -> w316
              frame #0 {
                n129 = local read "Offset_rueda WS 1"() -> (w366:fxp<+/-,24,-4>)
                n130 = local read "Offset_rueda WS 2"() -> (w367:fxp<+/-,24,-4>)
                n131 = local read "Frecuencia de muestreo (Hz)"() -> (w381:dbl)
                n132 = local read "Escaneos de la FIFO por canal"() -> (w370:u32)
                n133 = local read "Canal cero WS1?"() -> (w375:bool)
                n134 = local read "Count(mSec)"() -> (w374:u32)
                n135 = local read "Frecuencia de muestreo y módulo CRIO"() -> (w377:T3)
                n136 = local read "Canal cero WS2"() -> (w365:bool)
                n137 = local read "Digital?"() -> (w376:bool)
                n138 = Get Date/Time In Seconds() -> (seconds since 1Jan1904=→"Inicio pasada":timestamp)
                n139 = local read "Nº de acelerómetros"() -> (w363:i32)
                n140 = local read "Nº inductivos"() -> (w364:i32)
                n141 = local write "TAGs"(string[] [] ("TAGs")) -> ()
                n142 = xnode "Read/Write Control"("FPGA VI Reference In"=w390, "error in"=w389, "Data Rate"=w377, "Digital?"=w376, "Canal cero WS1?"=w375, "Count(mSec)"=w374, "Offset_WS1"=w366, "Offset_WS2"=w367, "Canal cero WS2?"=w365) -> ("FPGA VI Reference Out"=w380:refnum<k20>, "error out"=w379:errorcluster)
                n143 = local read "RFID LR6 on?"() -> (w368:bool)
                n144 = Add(x=w364, y=w363) -> (x+y=w369:i32)
                n145 = case shown="False" w368 {
                  tunnel: [errorcluster {"status"=FALSE, "code"=0, "source"=""} ("error out") w395] -> w373
                  frame False {
                  }
                  frame True {
                    n146 = local read "RFID_LR6_Error"() -> (w396:errorcluster)
                    n147 = call "LH6HD.vi"("error in (no error)"=w396, "Action"=enum16{"Init", "Start", "Read", "Stop", "Exit"}."Start") -> ("error out"=w395:errorcluster)  [unwired: 8 in, 1 out]
                  }
                }
                n148 = call "DMACalc.vi"("Number of Channels"=w369, "Number of Samples"=w370, "Rate (Hz)"=w381) -> ("Block Size"=w385:u32, "Time to Acquire Block (ms)"=w386:i32, "Host Buffer Size"=w391:u32)  [unwired: 6 in]
                n149 = call "Pathhorafech(SubVI)_varios.vi"("Folder path"=path "c:/Trenes", "Nº de acelerómetros"=w363, "Nº inductivos"=w364) -> ("Acel_Paths"=w359:path[])  [unwired: 1 in, 1 out]
                "Nombre de archivo" <- w359
                n150 = Index Array(array=w359) -> (element=w358:path)  [unwired: 1 in]
                n151 = for {
                  tunnel: w359 -> [w400] mode=indexing
                  tunnel: [w399] -> w384 mode=indexing
                  tunnel: [w398] -> w383
                  n152 = Open/Create/Replace File(file path (use dialog)=w400, operation (0:open)=T5."replace or create", access (0:read/write)=enum16{"read/write", "read-only", "write-only"}."read/write", disable buffering (F)=TRUE) -> (refnum out=w399:refnum<file>, error out=w398:errorcluster)  [unwired: 1 in, 2 out]
                }
                n153 = xnode "Invoke Method"("FPGA VI Reference In"=w380, "error in"=w379, "Requested Depth"=w391) -> ("FPGA VI Reference Out"=w393:refnum<k20>, "error out"=w392:errorcluster)  [unwired: 1 out]
                n154 = local read "Report"() -> (w362:string)
                n155 = Path To String(path=w358) -> (string=w356:string)
                n156 = Concatenate Strings("\nFile created: ", w356, "\n", w362) -> (w361:string)
                n157 = xnode "Invoke Method"("FPGA VI Reference In"=w393, "error in"=w392) -> ("FPGA VI Reference Out"=w388:refnum<k20>, "error out"=w387:errorcluster)
                n158 = local write "Report"(w361) -> ()
              }
              frame #1 {
                n159 = while "Data Acquisition" {
                  tunnel: w419 -> [w473]
                  shift-right: [w497] -> _
                  shift-left: u32 0 ("t") -> [w493]
                  tunnel: w417 -> [w498]
                  tunnel: w416 -> [w496]
                  shift-right: [w499] -> w421
                  shift-left: w418 -> [w490]
                  tunnel: [w494] -> w422
                  tunnel: w415 -> [w477]
                  tunnel: [w478] -> w420
                  shift-right: [w476] -> w413
                  shift-left: w414 -> [w486]
                  stop <- w495 stop-if-true
                  # "Detector de presencia"
                  # "Mide el tiempo de paso del tren y con ello se puede calcular\nla velocidad la unidad"
                  n160 = xnode "Invoke Method"("FPGA VI Reference In"=w473, "error in"=w490, "Number of Elements"=w493, "Timeout (ms)"=0) -> ("FPGA VI Reference Out"=w470:refnum<k20>, "error out"=w475:errorcluster, "Data"=w489:fxp<+/-,24,4>[], "Elements Remaining"=w491:u32)
                  n161 = case "Data Ready" shown="Default" w493 {
                    tunnel: w498 -> [w521 _]
                    tunnel: [w520 u32 0 ("t")] -> w497
                    tunnel: w496 -> [w522 _]
                    tunnel: w491 -> [w519 _]
                    tunnel: w489 -> [_ w544]
                    tunnel: w486 -> [w518 w543]
                    tunnel: [w518 w545] -> w476
                    tunnel: w477 -> [w517 w542]
                    tunnel: [w517 w541] -> w478
                    frame 0 {
                      # "En este caso se compara los elementos que quedan\nen la FIFO del controlador con el tamaño dell bloque\nque aparece en el panel frontal. Si el número de \nelementos en la FIFO es mayor o igual que el tamaño\n del bloque se pasa al siguiente caso y se guardan \nlos datos en un archivo. El reloj que aparece es una\nespera para no consumir recursos."
                      n162 = Greater Or Equal?(x=w519, y=w522) -> (x >= y?=w523:bool)
                      n163 = case shown="False" w523 {
                        tunnel: [u32 0 ("Block Size") w527] -> w520
                        tunnel: [w526 0 ("t")] -> w524
                        tunnel: w521 -> [w526 _]
                        tunnel: w522 -> [_ w527]
                        frame False {
                        }
                        frame True {
                        }
                      }
                      n164 = call "WaitMinTimeBetweenCall.vi"("Minimum ms between calls"=w524) -> ()  [unwired: 2 in]
                    }
                    frame Default {
                      n165 = To Single Precision Float(number=w544) -> (single precision float=w531:sgl[])
                      n166 = Decimate 1D Array(w531) -> (w537:sgl[], w540:sgl[], w539:sgl[], w538:sgl[], w536:sgl[], w535:sgl[], w534:sgl[], w533:sgl[], w532:sgl[], w529:sgl[])
                      n167 = Build Array(w537, w540, w539, w538, w536, w535, w534, w533, w532, w529) -> (w530:sgl[][])
                      n168 = for {
                        tunnel: T6."little-endian" ("byte order (0:big-endian, network order)") -> [w554]
                        shift-right: [w548] -> w545
                        shift-left: w543 -> [w549]
                        tunnel: w530 -> [w552] mode=indexing
                        tunnel: w542 -> [w551] mode=indexing
                        tunnel: [w550] -> w541 mode=indexing
                        n169 = Write to Binary File(file (use dialog)=w551, data=w552, error in=w549, 5:FALSE ("prepend array or string size? (T)"), 9:w554) -> (refnum out=w550:refnum<file>, error out=w548:errorcluster)  [unwired: 2 out]
                      }
                    }
                  }
                  n170 = xnode "Read/Write Control"("FPGA VI Reference In"=w470, "error in"=w475) -> ("FPGA VI Reference Out"=w488:refnum<k20>, "error out"=w487:errorcluster, "Parar"=w466:bool, "Nº Ruedas 1"=→"Nº Ruedas 1":i32, "NºRuedas 2"=→"NºRuedas 2":i32)
                  "Parar" <- w466
                  n171 = case shown="False" w466 {
                    tunnel: [w504 w512] -> w467
                    tunnel: [w505 0.0] -> w481
                    frame False {
                      n172 = local read "Inicio pasada"() -> (w508:timestamp)
                      n173 = Get Date/Time In Seconds() -> (seconds since 1Jan1904=w507:timestamp)
                      n174 = local read "Tiempo de adquisicion"() -> (w500:dbl)
                      n175 = To Double Precision Float(number=w507) -> (double precision float=w506:dbl)
                      n176 = To Double Precision Float(number=w508) -> (double precision float=w509:dbl)
                      n177 = Subtract(x=w506, y=w509) -> (x-y=w505:dbl)
                      "Tiempo de paso (s)" <- w505
                      n178 = local write "Tiempo"(w506) -> ()
                      n179 = local read "Boton Adquirir?"() -> (w501:bool)
                      n180 = Greater?(x=w505, y=w500) -> (0:w503:bool)
                      n181 = Select(t=w503, s=w501, f=FALSE) -> (s? t:f=w504:bool)
                    }
                    frame True {
                      n182 = local read "Tiempo"() -> (w516:dbl)
                      n183 = local read "Tiempo extra al detector de paso (s)"() -> (w511:dbl)
                      n184 = Get Date/Time In Seconds() -> (seconds since 1Jan1904=w513:timestamp)
                      n185 = To Double Precision Float(number=w513) -> (double precision float=w514:dbl)
                      n186 = Subtract(x=w514, y=w516) -> (x-y=w515:dbl)
                      n187 = Greater?(x=w515, y=w511) -> (0:w512:bool)
                    }
                  }
                  "Fin" <- w467
                  n188 = local read "Timeout ruedas"() -> (w465:dbl)
                  n189 = xnode ("CheckLate")("FPGA VI Reference In"=w488, "error in"=w487) -> ("FPGA VI Reference Out"=w472:refnum<k20>, "error out"=w483:errorcluster, "Buffer Underflow"=→"Buffer Underflow":bool, "Buffer Overflow"=w474:bool)
                  "Buffer Overflow" <- w474
                  n190 = Greater?(x=w481, y=w465) -> (0:w479:bool)
                  "Timeout ruedas" <- w479
                  n191 = call "ErrorOverFlow.vi"("Buffer Overflow"=w474) -> ("error out"=w482:errorcluster)
                  n192 = Merge Errors(w483, w482) -> (w471:errorcluster)
                  n193 = Unbundle By Name(w476) -> ("status"=w480:bool)
                  n194 = Unbundle By Name(w471) -> ("status"=w485:bool)
                  n195 = Compound Arithmetic op=OR(w485, w467, w479, w480) -> (w495:bool)
                  "result" <- w495
                  n196 = case "Flush" shown="True" w495 {
                    tunnel: [w555 w560] -> w499
                    tunnel: [w556 w559] -> w494
                    tunnel: w472 -> [w556 w558]
                    tunnel: w471 -> [w555 w557]
                    frame False {
                    }
                    frame True {
                      n197 = xnode "Invoke Method"("FPGA VI Reference In"=w558, "error in"=w557) -> ("FPGA VI Reference Out"=w559:refnum<k20>, "error out"=w560:errorcluster)
                    }
                  }
                  "Block Size" <- w496
                  "Time to Acquire Block (ms)" <- w498
                }
                n198 = call <vilib>:"Watchdog Whack.vi"("error in (no error)"=w408, "reset watchdog after expire? (F)"=TRUE, "watchdogID in"=w409) -> ("error out"=w405:errorcluster, "watchdogID out"=w406:u64)  [unwired: 2 in, 1 out]
                n199 = local read "RFID LR6 on?"() -> (w404:bool)
                n200 = case shown="True" w404 {
                  tunnel: w411 -> [w423 w429]
                  tunnel: [w423 w428] -> w410
                  frame False {
                  }
                  frame True {
                    n201 = while {
                      shift-right: [w436] -> w428
                      shift-left: w429 -> [w437]
                      shift-right: [w435] -> w426
                      shift-left: string[] [] -> [w434]
                      shift-right: [w430] -> w424
                      shift-left: i32[] [] -> [w431]
                      i -> [w432]
                      stop <- w433 stop-if-true
                      n202 = case shown="No Error" w437 {
                        selector: w437 -> [w448 _]
                        tunnel: [w447 w463] -> w436
                        tunnel: [w443 string[] []] -> w435
                        tunnel: w434 -> [w442 _]
                        tunnel: w432 -> [w441 _]
                        tunnel: w431 -> [w440 _]
                        tunnel: [w439 i32[] []] -> w430
                        frame No Error {
                          n203 = call "LH6HD.vi"("error in (no error)"=w448, "Action"=enum16{"Init", "Start", "Read", "Stop", "Exit"}."Read") -> ("error out"=w447:errorcluster, "Tag"=w444:string)  [unwired: 8 in]
                          n204 = Not Equal?(x="", y=w444) -> (x != y?=w445:bool)
                          n205 = case shown="False" w445 {
                            tunnel: w444 -> [_ w457]
                            tunnel: [w451 w456] -> w443
                            tunnel: w442 -> [w451 w455]
                            tunnel: w441 -> [_ w452]
                            tunnel: w440 -> [w450 w454]
                            tunnel: [w450 w453] -> w439
                            frame False {
                            }
                            frame True {
                              n206 = Build Array (concatenate)(w455, w457) -> (w456:string[])
                              n207 = Build Array (concatenate)(w454, w452) -> (w453:i32[])
                            }
                          }
                        }
                        frame Error {
                          n208 = local read "LR6 IP address"() -> (w460:string)
                          n209 = local read "DeviceAddress"() -> (w458:u8)
                          n210 = local read "Port LR6"() -> (w461:u16)
                          n211 = call "LH6HD.vi"("DeviceAddress"=w458, "Reader Port"=w461, "IP Address"=w460, "Action"=enum16{"Init", "Start", "Read", "Stop", "Exit"}."Init") -> ("error out"=w463:errorcluster)  [unwired: 6 in, 1 out]
                        }
                      }
                      n212 = Wait Until Next ms Multiple(millisecond multiple=u32 500) -> ()  [unwired: 1 out]
                      n213 = local read "result"() -> (w433:bool)
                      "it-LR6" <- w432
                    }
                    "TAGs LR6" <- w426
                    "it-read-LR6" <- w424
                  }
                }
              }
              frame #2 {
                # "ORGANIZAR\nTAGS AQUÍ"
                n214 = local read "RFID LR6 on?"() -> (w589:bool)
                n215 = local read "RFID NEM on?"() -> (w590:bool)
                n216 = Array Size(array=w603) -> (size(s)=w601:i32)
                n217 = case shown="False" w589 {
                  tunnel: w599 -> [w633 w639]
                  tunnel: [w633 w634] -> w598
                  frame False {
                  }
                  frame True {
                    n218 = call "LH6HD.vi"("error in (no error)"=w639, "Action"=enum16{"Init", "Start", "Read", "Stop", "Exit"}."Stop") -> ("error out"=w634:errorcluster)  [unwired: 8 in, 1 out]
                    n219 = call "Reporting_error.vi"("error out 2"=w634, "Concept"="Active RFID") -> ("Reporting"=w636:string)  [unwired: 1 in]
                    n220 = local read "Report"() -> (w637:string)
                    n221 = Concatenate Strings(w636, w637) -> (w635:string)
                    n222 = local write "Report"(w635) -> ()
                  }
                }
                n223 = local read "TAGs LR6"() -> (w569:string[])
                n224 = local read "AURA wheel test"() -> (w568:bool)
                n225 = Decrement(x=w601) -> (x-1=w602:i32)
                n226 = case shown="True" w590 {
                  tunnel: [string[] [] ("TagArray") w646] -> w572
                  tunnel: [cluster{"TagCode":string, "FirstSeemUs":u64}[] [] ("TagData out") w645] -> w571
                  frame False {
                  }
                  frame True {
                    n227 = call "IF2_TagBuffer.vi"("Action"=enum16{"Init", "WriteTagData", "ReadTagData"}."ReadTagData") -> ("error out"=w644:errorcluster, "TagData out"=w645:cluster{"TagCode":string, "FirstSeemUs":u64}[])  [unwired: 9 in]
                    n228 = local read "connection ID"() -> (w643:refnum<k5>)
                    n229 = call "RFID_TAGS_Sort.vi"("TagData in"=w645) -> ("TagString"=w647:string, "TagArray"=w646:string[])  [unwired: 9 in]
                    n230 = call "IF2_Clear_buffer.vi"("error in (no error)"=w644, "TCP Network Connection in"=w643) -> ()  [unwired: 8 in, 2 out]
                    n231 = call "Reporting_error.vi"("error out 2"=w644, "Concept explanation"=w647, "Concept"="Passive RFID") -> ("Reporting"=w650:string)
                    n232 = local read "Report"() -> (w651:string)
                    n233 = Concatenate Strings(w650, w651) -> (w649:string)
                    n234 = local write "Report"(w649) -> ()
                  }
                }
                "TAGs HEX" <- w572
                "TagData out" <- w571
                n235 = Index Array(array=w603, index=w602) -> (element=w611:refnum<file>)
                n236 = local write "result"(FALSE ("result")) -> ()
                n237 = xnode "Read/Write Control"("FPGA VI Reference In"=w588, "error in"=w587) -> ("FPGA VI Reference Out"=w624:refnum<k20>, "error out"=w585:errorcluster, "Chassis Temperature"=w632:i16)
                n238 = Select(t=w569, s=w568, f=string[] ["A0000000000000000TESTNEM700", "A0000000000000000TESTNEM800"]) -> (s? t:f=w573:string[])
                n239 = Divide(x=w632, y=4.0) -> (x/y=w582:dbl)
                "Temperatura (ºC)" <- w582
                n240 = local read "Tiempo de paso (s)"() -> (w622:dbl)
                n241 = for {
                  tunnel: w573 -> [w653] mode=indexing
                  tunnel: [w653] -> w561 mode=indexing
                }
                n242 = local write "RFID_LR6_Error"(w598) -> ()
                n243 = Index Array(array=w572) -> (element=w597:string)  [unwired: 1 in]
                n244 = local read "Nº Ruedas 1"() -> (w580:i32)
                n245 = local read "NºRuedas 2"() -> (w583:i32)
                n246 = Not Equal?(x=w597, y="" ("delimiter (\\t)")) -> (x != y?=w595:bool)
                "Plataformas?" <- w595
                n247 = Multiply(x=w622, y=1000.0) -> (x*y=w581:dbl)
                n248 = case shown="True" w595 {
                  tunnel: w561 -> [w654 _]
                  tunnel: [w654 w655] -> w565
                  tunnel: w571 -> [_ w656]
                  tunnel: w572 -> [_ _]
                  frame False {
                  }
                  frame True {
                    n249 = local read "Tiempo de paso (s)"() -> (w660:dbl)
                    n250 = local read "Tabla_flota"() -> (w658:string[][])
                    n251 = local read "Inicio pasada"() -> (w659:timestamp)
                    n252 = local read "RFID_status"() -> (w657:path)
                    n253 = call "TagNormalizaction.vi"("Inicio pasada"=w659, "Tiempo de paso (s)"=w660, "TagData in"=w656, "Tabla_flota"=w658) -> ("Normalized Tags"=w655:string[])  [unwired: 5 in, 2 out]
                    n254 = call "write_tag_status.vi"("Inicio pasada"=w659, "Tabla_flota"=w658, "file path (use dialog)"=w657) -> ()  [unwired: 8 in]
                  }
                }
                "TAGs" <- w565
                n255 = Build Array(w582, w581, w580, w583) -> (w584:dbl[])
                n256 = Build Array(w582, w581, w580) -> (w579:dbl[])
                n257 = local read "Direccion 0?"() -> (w578:bool)
                n258 = local read "Nombre de archivo"() -> (w610:path[])
                n259 = Bundle("error out"=w585, w584, "Normalized Tags"=w565, "Direccion 0?"=w578) -> (w577:T11)  [unwired: 1 in]
                n260 = for {
                  shift-right: [w666] -> w616
                  shift-left: string[] [] -> [w665]
                  tunnel: w565 -> [w664] mode=indexing
                  n261 = Insert Into Array(array=w665, new element=w664) -> (w666:string[])  [unwired: 1 in]
                }
                n262 = xnode "Read/Write Control"("FPGA VI Reference In"=w624, "error in"=w585, "Stop"=TRUE ("stop")) -> ("FPGA VI Reference Out"=w613:refnum<k20>, "error out"=w612:errorcluster)
                n263 = call "Reporting_acqu.vi"("output cluster"=w577, "address repoting"=path "C:/Reporting/Reporting_adqu.txt" ("file (use dialog)")) -> ("Reporting"=w574:string)  [unwired: 1 in]
                n264 = Delete From Array(array=w610) -> (deleted portion=w609:path)  [unwired: 2 in, 1 out]
                n265 = local read "Report"() -> (w575:string)
                n266 = To Single Precision Float(number=w579) -> (single precision float=w630:sgl[])
                n267 = Array Subset(array=w565, index=0) -> (w566:string[])  [unwired: 1 in]
                n268 = Array Subset(array=w565, index=2) -> (w567:string[])  [unwired: 1 in]
                n269 = Path To String(path=w609) -> (string=w615:string)
                n270 = Concatenate Strings(w574, w575) -> (w576:string)
                n271 = Write to Binary File(file (use dialog)=w611, data=w630, error in=w627, 5:FALSE ("prepend array or string size? (T)"), 9:T6."little-endian" ("byte order (0:big-endian, network order)")) -> (error out=w608:errorcluster)  [unwired: 3 out]
                n272 = xnode "Invoke Method"("FPGA VI Reference In"=w613, "error in"=w612) -> ("FPGA VI Reference Out"=w620:refnum<k20>, "error out"=w619:errorcluster)
                n273 = local read "Timeout ruedas"() -> (w623:bool)
                n274 = local write "Report"(w576) -> ()
                n275 = Build Array(w566, w567) -> (→"appended array":string[][])
                n276 = Build Array (concatenate)(w615, w616) -> (w593:string[])
                n277 = local read "TAGS leidos"() -> (w604:path)
                n278 = for {
                  shift-right: [w663] -> w618
                  shift-left: w608 -> [w662]
                  tunnel: w603 -> [w661] mode=indexing
                  n279 = Close File(refnum=w661, error in=w662) -> (error out=w663:errorcluster)  [unwired: 1 out]
                }
                n280 = call-poly <vilib>:"Write Delimited Spreadsheet.vi"("file path (dialog if empty)"=w604, "1D data"=w593, "append to file? (F)"=TRUE ("transpose? (no:F)"), "transpose? (F)"=TRUE ("append to file? (new file:F)"), "delimiter (\\t)"=";" ("delimiter (\\t)")) -> ()  [unwired: 9 in, 2 out]
                n281 = Select(t="TEST", s=w623, f="Procesado") -> (s? t:f=w625:string)
              }
            }
            n282 = call <vilib>:"Watchdog Clear.vi"("error in (no error)"=w316, "watchdogID in"=w317) -> ("error out"=w318:errorcluster)  [unwired: 5 in]
            n283 = Merge Errors(w341, w318) -> (w340:errorcluster)
            n284 = Unbundle By Name(w343) -> ("status"=w332:bool)
            n285 = Unbundle By Name(w341) -> ("status"=w333:bool)
            n286 = Compound Arithmetic op=OR(w332, w333) -> (w330:bool)
            n287 = Select(t="TEST", s=w330, f=w331) -> (s? t:f=w328:string)
          }
          frame "Procesado" {
            n288 = local read "Watchdog config"() -> (w678:T2)
            n289 = flat-sequence {
              tunnel: w672 -> [w691]
              tunnel: [w691] -> w671
              tunnel: w670 -> [w687]
              tunnel: [w687] -> w669
              frame #0 {
                n290 = local read "Report"() -> (w688:string)
                n291 = call "Reporting_datetime.vi"() -> ("String"=w686:string)  [unwired: 11 in]
                n292 = Concatenate Strings(w686, "\nSTATUS: PROCESSING\nProcessing the measurement\n\n", w688) -> (w690:string)
                n293 = local write "Report"(w690) -> ()
              }
            }
            n294 = call <vilib>:"Watchdog Configure.vi"("error in (no error)"=w681, "expiration actions"=w678, "timeout (1 sec)"=300.0) -> ("error out"=w680:errorcluster, "watchdogID"=w677:u64)  [unwired: 1 in, 2 out]
            n295 = flat-sequence {
              tunnel: w680 -> [w698]
              tunnel: w677 -> [w694]
              tunnel: [w693] -> w676
              tunnel: [w692] -> w675
              tunnel: [w910] -> w674
              tunnel: w676 -> [w910]
              tunnel: [w909] -> w673
              tunnel: w675 -> [w909]
              frame #0 {
                n296 = flat-sequence {
                  tunnel: [w771] -> w700
                  tunnel: [w757] -> w699
                  tunnel: w698 -> [w741]
                  tunnel: [w724] -> w695
                  tunnel: [w759] -> w697
                  tunnel: [w716] -> w696
                  tunnel: w694 -> [w742]
                  tunnel: [w739] -> w693
                  tunnel: [w738] -> w692
                  frame #0 {
                    # "Se cambia la variable Tags, por TagDaata out"
                    n297 = local read "AURA wheel test"() -> (w714:bool)
                    n298 = case shown="True" w714 {
                      tunnel: [w773 w775] -> w703
                      tunnel: [w774 path[] [path "c:/Trenes_prueba/A_0_TEST.bin", path "c:/Trenes_prueba/A_1_TEST.bin", path "c:/Trenes_prueba/A_2_TEST.bin", path "c:/Trenes_prueba/A_3_TEST.bin", path "c:/Trenes_prueba/A_4_TEST.bin", path "c:/Trenes_prueba/A_5_TEST.bin", path "c:/Trenes_prueba/A_6_TEST.bin", path "c:/Trenes_prueba/A_7_TEST.bin", path "c:/Trenes_prueba/I_0_TEST.bin", path "c:/Trenes_prueba/I_1_TEST.bin"]] -> w713
                      frame False {
                        n299 = local read "Nombre de archivo"() -> (w774:path[])
                        n300 = local read "TAGs"() -> (w773:string[])
                      }
                      frame True {
                        w775 = string[] ["A0000000000000000TESTNEM700", "A0000000000000000TESTNEM800"]
                        n301 = local write "TAGs LR6"(w775) -> ()
                      }
                    }
                    n302 = local read "Tabla_flota"() -> (w756:string[][])
                    n303 = call <vilib>:"Watchdog Whack.vi"("error in (no error)"=w741, "reset watchdog after expire? (F)"=TRUE, "watchdogID in"=w742) -> ("error out"=w738:errorcluster, "watchdogID out"=w739:u64)  [unwired: 2 in, 1 out]
                    n304 = local read "Puntos medios de las ventanas"() -> (w758:dbl[][])
                    n305 = call "Series_ejes_flota.vi"("Tabla_flota"=w756, "Tags"=w703) -> ("Nº Ejes"=w706:i32[], "Series del convoy"=w707:string[])  [unwired: 2 in, 1 out]
                    n306 = Array Size(array=w713) -> (size(s)=w765:i32)
                    n307 = Array Size(array=w707) -> ()  [unwired: 1 out]
                    n308 = Subtract(x=w765, y=2 ("length")) -> (x-y=w767:i32)
                    n309 = Add Array Elements(numeric array=w706) -> (sum=w705:i32)
                    n310 = local read "Series_flota"() -> (w755:string[])
                    n311 = Delete From Array(array=w713, length=2, index=w767) -> (deleted portion=w743:path[], array with subset deleted=w759:path[])
                    n312 = local read "date/time string"() -> (w704:string)
                    n313 = Index Array(array=w743) -> (element #2=w737:path)  [unwired: 2 in, 1 out]
                    n314 = call "Distancias_ejes_convoy.vi"("Series_flota1"=w707, "Ejes_UT"=w706, "Puntos medios de las ventanas"=w758, "Series_flota"=w755) -> ("Distancias_entre_ejes_convoy"=w757:dbl[])  [unwired: 1 in]
                    n315 = Read from Binary File(5:sgl 0.0, 9:T6."little-endian" ("byte order (0:big-endian, network order)"), 10:-1 ("count (1)"), 11:w737) -> (0:w763:errorcluster, 2:w745:sgl[], 3:w764:refnum<file>)  [unwired: 1 in, 2 out]
                    n316 = local read "Frecuencia de muestreo (Hz)"() -> (w728:dbl)
                    n317 = local read "appended array"() -> (w701:string[][])
                    n318 = local read "Offset_rueda WS 2"() -> (w729:fxp<+/-,24,-4>)
                    n319 = local read "it-LR6"() -> (w748:i32)
                    n320 = local read "it-read-LR6"() -> (w749:i32[])
                    n321 = local read "Plataformas?"() -> (w747:bool)
                    n322 = local read "TAGs LR6"() -> (w750:string[])
                    n323 = Close File(refnum=w764, error in=w763) -> (error out=w709:errorcluster)  [unwired: 1 out]
                    n324 = local read "TAGs HEX"() -> (w702:string[])
                    n325 = Array Size(array=w745) -> (size(s)=w754:i32)
                    n326 = Subtract(x=w754, y=3 ("length")) -> (x-y=w752:i32)
                    n327 = Delete From Array(array=w745, length=3, index=w752) -> (array with subset deleted=w735:sgl[])  [unwired: 1 out]
                    n328 = call "TAGs_AURAwheel_TAGM_NEM.vi"("Nº Ejes"=w706, "TAGs"=w703, "Ejes_convoy"=w705, "it-LR6"=w748, "TAGs LR6"=w750, "it-read-LR6"=w749, "Plataformas?"=w747) -> ("TAGS_AURA"=→"TAGs_AURAwheel":string[][])  [unwired: 1 in]
                    n329 = call "Analogico_digital.vi"("Array"=w735, "Offset WS"=w729, "Frecuencia muestreo"=w728) -> ("array w/ subset deleted"=w730:sgl[], "Tiempo\npaso"=w727:dbl)  [unwired: 6 in]
                    n330 = call "a.vi"("string"=w704, "TAGs 2"=w703, "string 4"=w701, "string 3"=w702) -> ()  [unwired: 8 in]
                    n331 = call "Puntos medio de pulso.vi"("DI Inductivo"=w730) -> ("Puntos"=w771:sgl[], "Número de ejes"=w718:i32)  [unwired: 1 in]
                    "Número de ejes detectados" <- w718
                    n332 = disable-structure shown="Enabled" {
                      disable-tunnel: w735 -> [w783 w786]
                      disable-tunnel: [FALSE ("element") TRUE ("element")] -> w732
                      disable-tunnel: [w777 w785] -> w731
                      frame Disabled {
                        n333 = Equal?(x=w783, y=0.0) -> (x = y?=w780:bool[])
                        n334 = Equal?(x=w783, y=1.0) -> (x = y?=w781:bool[])
                        n335 = Or(x=w780, y=w781) -> (x .or. y?=w777:bool[])
                      }
                      frame Enabled {
                        n336 = Greater?(x=w786, y=0.1) -> (0:w785:bool[])
                      }
                    }
                    n337 = Decrement(x=w718) -> (x-1=w770:i32)
                    n338 = call "Reporting_error.vi"("error out 2"=w709, "Concept"="Measurement reading") -> ("Reporting"=w711:string)  [unwired: 1 in]
                    n339 = Get Volume Info(11:path "c:/" ("path")) -> (1:w719:i64)  [unwired: 1 in, 5 out]
                    "Disco Duro Disponible (bytes)" <- w719
                    n340 = local read "Report"() -> (w712:string)
                    n341 = call "Calculo_Velocidad.vi"("Tiempo de paso (s)"=w727, "Ejes"=w770, "Puntos iniciales de las ventanas"=w757) -> ("V (m/s)"=→"V (m/s)":dbl, "Longitud de la unidad"=→"Longitud de la unidad":dbl)
                    n342 = Concatenate Strings(w711, w712) -> (w710:string)
                    n343 = Equal?(x=w705, y=w718) -> (x = y?=w716:bool)
                    n344 = Not Equal?(x=w718, y=0) -> (x != y?=w715:bool)
                    n345 = Search 1D Array(1D array=w731, element=w732) -> (index of element=w733:i32)  [unwired: 1 in]
                    n346 = local write "Report"(w710) -> ()
                    n347 = Build Array(w705, w718, w719) -> (w723:i64[])
                    n348 = Equal?(x=w733, y=-1) -> (x = y?=w736:bool)
                    n349 = Compound Arithmetic op=AND(w716, w715, w736) -> (w724:bool)
                    "Archivo\nvalido?" <- w724
                    n350 = Bundle(w723, w724) -> (w721:cluster{i64[], bool})  [unwired: 1 in]
                    n351 = call "Reporting_proc.vi"("output cluster 2"=w721, "address repoting"=path "C:/Reporting/Reporting_proc.txt" ("file (use dialog)")) -> ("Reporting"=w720:string)  [unwired: 1 in]
                    n352 = local read "Report"() -> (w725:string)
                    n353 = Concatenate Strings(w720, w725) -> (w726:string)
                    n354 = local write "Report"(w726) -> ()
                  }
                }
                n355 = case shown="True" w695 {
                  tunnel: w700 -> [_ w821]
                  tunnel: w699 -> [_ w819]
                  tunnel: w697 -> [_ w820]
                  tunnel: w696 -> [w788 _]
                  frame False {
                    n356 = local read "Nombre de archivo"() -> (w789:path[])
                    n357 = for {
                      tunnel: w789 -> [w791] mode=indexing
                      tunnel: w788 -> [w790]
                      n358 = flat-sequence {
                        tunnel: w791 -> [w801]
                        tunnel: [w801] -> w794
                        tunnel: [w800] -> w793
                        tunnel: w790 -> [w799]
                        tunnel: w794 -> [w808]
                        tunnel: [w807] -> w792
                        tunnel: w793 -> [w807]
                        tunnel: w792 -> [w810]
                        frame #0 {
                          w800 = path "c:/Est_Adq.csv" ("file path (use dialog)")
                          n359 = Path To String(path=w801) -> (string=w802:string)
                          n360 = Select(t="Nº Ejes detectados WS diferente a Nº Ejes TAGs" ("delimiter (\\t)"), s=w799, f="La señal del inductivo no es digital" ("delimiter (\\t)")) -> (s? t:f=w796:string)
                          n361 = Build Array(w802, w796) -> (w795:string[])
                          n362 = call-poly <vilib>:"Write Delimited Spreadsheet.vi"("file path (dialog if empty)"=w800, "1D data"=w795, "append to file? (F)"=FALSE ("transpose? (no:F)"), "transpose? (F)"=TRUE ("append to file? (new file:F)"), "delimiter (\\t)"=";" ("delimiter (\\t)")) -> ()  [unwired: 9 in, 2 out]
                        }
                        frame #1 {
                          n363 = local read "Borrar archivos\nadquisicion con error"() -> (w806:bool)
                          n364 = case shown="True" w806 {
                            tunnel: w808 -> [_ w809]
                            frame False {
                            }
                            frame True {
                              n365 = Delete(path (use dialog)=w809) -> ()  [unwired: 1 in, 6 out]
                            }
                          }
                        }
                        frame #2 {
                          n366 = File/Directory Info(path=w810) -> (size=w813:i64)  [unwired: 1 in, 6 out]
                          n367 = Greater?(x=w813, y=i64 1000000) -> (0:w811:bool)
                          n368 = case shown="True" w811 {
                            tunnel: w810 -> [_ w814]
                            frame False {
                            }
                            frame True {
                              n369 = Delete(path (use dialog)=w814) -> ()  [unwired: 4 in, 3 out]
                            }
                          }
                        }
                      }
                    }
                  }
                  frame True {
                    n370 = flat-sequence {
                      tunnel: w821 -> [w898]
                      tunnel: w820 -> [w895]
                      tunnel: w819 -> [w899]
                      tunnel: [w882] -> w818
                      frame #0 {
                        # "SALIDA \n\nMáximos por rueda inductivo"
                        # "8 acelerómetros"
                        # "Velocidad"
                        n371 = local read "Frecuencia de muestreo (Hz)"() -> (w897:dbl)
                        n372 = local read "Distancia de acelerómetros"() -> (w887:dbl[])
                        n373 = local read "Parámetros acelerómetros"() -> (w894:dbl[])
                        n374 = local read "Número de ejes detectados"() -> (w893:i32)
                        n375 = local read "Distancias generales"() -> (w892:dbl[])
                        n376 = local read "dt RMS"() -> (w896:dbl)
                        n377 = local read "Direccion 0?"() -> (w884:bool)
                        n378 = Index Array(array=w892, index=1) -> (element=w890:dbl)
                        n379 = Select(t=0.0, s=w884, f=w890) -> (s? t:f=w888:dbl)
                        n380 = Subtract(x=w888, y=w887) -> (x-y=w886:dbl[])
                        n381 = Absolute Value(x=w886) -> (abs(x)=w885:dbl[])
                        n382 = call "Procesado_aRMS_BIdirecc.vi"("Paths_canales_aRMS"=w895, "Ejes Procesados"=w893, "Distancias\nacelerometros"=w885, "Distancias generales (m)"=w892, "Distancias centrales de las ruedas\n               configuración (m)"=w899, "Frecuencia de muestreo"=w897, "Parámetros acelerómetros"=w894, "dt RMS 2"=w896, "Puntos"=w898) -> ("Max RMS Ruedas"=w883:dbl[][])  [unwired: 2 in]
                        n383 = Transpose 2D Array(2D array=w883) -> (transposed array=w882:dbl[][])
                        "Max RMS Ruedas" <- w882
                        n384 = call "Reporting_proc_RMS.vi"("Max RMS Ruedas"=w882) -> ("String"=w880:string)
                        n385 = local read "Report"() -> (w881:string)
                        n386 = Concatenate Strings(w880, w881) -> (w879:string)
                        n387 = local write "Report"(w879) -> ()
                      }
                    }
                    n388 = local read "Use Aura?"() -> (w817:bool)
                    n389 = local read "TAGs_AURAwheel"() -> (w816:string[][])
                    n390 = local read "Nº Ejes"() -> (w815:i32[])
                    n391 = for {
                      tunnel: w817 -> [w825]
                      tunnel: w816 -> [w824] mode=indexing
                      shift-right: [w823] -> _
                      shift-left: w818 -> [w826]
                      tunnel: w815 -> [w822] mode=indexing
                      # "dev.api.aurawheel.com"
                      n392 = case shown="True" w825 {
                        tunnel: w826 -> [w827 w846]
                        tunnel: w824 -> [_ w847]
                        tunnel: [w827 w845] -> w823
                        tunnel: w822 -> [_ w843]
                        frame False {
                        }
                        frame True {
                          w831 = "\n"
                          w854 = cluster{"status":string} {"status"=""}
                          n393 = local read "Parametros AuraWheel"() -> (w878:string[])
                          n394 = Delete From Array(array=w846, length=w843, index (row)=0) -> (deleted portion=w842:dbl[][], array with subset deleted=w845:dbl[][])  [unwired: 1 in]
                          n395 = Get Date/Time In Seconds() -> (seconds since 1Jan1904=w875:timestamp)
                          n396 = Format Date/Time String(time format string (%c)="%H:%M:%S%3u", seconds (now)=w875) -> (date/time string=w873:string)  [unwired: 1 in]
                          n397 = Get Date/Time In Seconds() -> (seconds since 1Jan1904=w850:timestamp)
                          n398 = Scan From String(format string="%d:%d:%f", input string=w873) -> (output 1=w870:i32, output 2=w869:i32, output 3=w867:dbl)  [unwired: 5 in, 3 out]
                          n399 = local read "V (m/s)"() -> (w838:dbl)
                          n400 = local read "Temperatura (ºC)"() -> (w848:dbl)
                          n401 = Multiply(x=w838, y=3.6) -> (x*y=w836:dbl)
                          n402 = Multiply(x=w867, y=1000.0) -> (x*y=w863:dbl)
                          n403 = call "Time_to_ms.vi"("seconds since 1Jan1904"=w850) -> ("Numeric"=w849:dbl)  [unwired: 1 in]
                          n404 = Multiply(x=w869, y=60000) -> (x*y=w864:i32)
                          n405 = Multiply(x=3600000, y=w870) -> (x*y=w865:i32)
                          n406 = Index Array(array=w878) -> (element #1=w841:string, element #2=w840:string, element #3=w839:string)  [unwired: 3 in]
                          n407 = call "aw_WRDCluster_8acel.vi"("Array TAGs"=w847, "Max RMS Ruedas"=w842, "TimeStamp"=w849, "p_sp"=w836, "p_tp"=w848) -> ("JSON cluster"=w876:T12)  [unwired: 1 in]
                          n408 = Compound Arithmetic op=ADD(w865, w864, w863) -> (w862:dbl)
                          n409 = To Variant(anything=w876) -> (Variant=w859:variant)
                          n410 = To Unsigned Long Integer(number=w862) -> (unsigned 32bit integer=w861:u32)
                          n411 = call "gjson_Create.vi"("JSON Object in"=w859) -> ("error out"=w857:errorcluster, "JSON String Out"=w858:string)  [unwired: 9 in]
                          n412 = Number To Decimal String(number=w861) -> (decimal integer string=w860:string)  [unwired: 1 in]
                          n413 = To Variant(anything=w854) -> (Variant=w853:variant)
                          n414 = call "aw_SendData.vi"("pwd"=w841, "x-nem-datetime"=w860, "User"=w840, "error in"=w857, "JSON Object"=w858, "URL"=w839) -> ("error out"=w855:errorcluster, "Response JSON"=w856:string, "Response headers"=w832:string)  [unwired: 3 in]
                          "Response headers" <- w832
                          n415 = call "gjson_Parse.vi"("error in"=w855, "JSON String In"=w856, "JSON Cluster"=w853) -> ("error out"=w851:errorcluster, "JSON Cluster Out"=w852:variant)  [unwired: 7 in]
                          n416 = Variant To Data(error in=w851, type=w854, Variant=w852) -> (data=→"data":cluster{"status":string}, error out=w833:errorcluster)
                          "error AURA" <- w833
                          n417 = local read "Report"() -> (w829:string)
                          n418 = call "Reporting_error.vi"("error out 2"=w833, "Concept"="A.U.R.A. Wheel Connection") -> ("Reporting"=w834:string)  [unwired: 1 in]
                          n419 = Concatenate Strings(w834, w831, w831, w832, w831) -> (w830:string)
                          "Report_AURA" <- w830
                          n420 = Concatenate Strings(w830, w829) -> (w828:string)
                          n421 = local write "Report"(w828) -> ()
                        }
                      }
                    }
                  }
                }
              }
              frame #1 {
                n422 = local read "Archivo\nvalido?"() -> (w906:bool)
                n423 = local read "Bytes libre despues de borrar"() -> (w907:u32)
                n424 = local read "Report_AURA"() -> (w903:string)
                n425 = local read "Max archivos"() -> (w904:u32)
                n426 = local read "Path LOG"() -> (w905:path)
                n427 = local read "LOG.txt"() -> (w900:path)
                n428 = local read "Report"() -> (w902:string)
                n429 = local read "Bytes min libre"() -> (w908:u32)
                n430 = local read "TAGS leidos"() -> (w911:path)
                n431 = File/Directory Info(path=w911) -> (size=w914:i64)  [unwired: 1 in, 6 out]
                n432 = case shown="True" w906 {
                  frame False {
                  }
                  frame True {
                    n433 = local read "Nombre de archivo"() -> (w916:path[])
                    n434 = call "Comprimir_a_1_archivo.vi"("Acel_paths"=w916) -> ("path_Pasada"=→"created path":path)
                  }
                }
                n435 = Greater?(x=w914, y=i64 1000000) -> (0:w912:bool)
                n436 = case shown="True" w912 {
                  tunnel: w911 -> [_ w917]
                  frame False {
                  }
                  frame True {
                    n437 = Delete(path (use dialog)=w917) -> ()  [unwired: 4 in, 3 out]
                  }
                }
                n438 = call "BORRADO_MEJORADO_Gonzalo.vi"("Bytes LIBRE OK"=w907, "Bytes Minimo de Memoria libre"=w908) -> ()  [unwired: 10 in]
                n439 = call "Saving_LOG.vi"("Path"=w900, "Report"=w902, "Report AURA"=w903, "Path Carpeta"=w905, "Nº Archivos Max"=w904) -> ("Report"=w901:string)  [unwired: 9 in, 1 out]
                n440 = local write "Report"(w901) -> ()
              }
            }
            n441 = call <vilib>:"Watchdog Clear.vi"("error in (no error)"=w673, "watchdogID in"=w674) -> ("error out"=w667:errorcluster)  [unwired: 5 in]
            n442 = Merge Errors(w669, w667) -> (w685:errorcluster)
            n443 = Unbundle By Name(w685) -> ("status"=w683:bool)
            n444 = Select(t="TEST", s=w683, f="Espera") -> (s? t:f=w682:string)
          }
          frame "TEST" {
            n445 = flat-sequence {
              tunnel: [w933] -> w920
              tunnel: w922 -> [w933]
              frame #0 {
                n446 = local read "Report"() -> (w934:string)
                n447 = call "Reporting_datetime.vi"() -> ("String"=w932:string)  [unwired: 11 in]
                n448 = Concatenate Strings(w932, "\nSTATUS: ERROR TEST\n\n", w934) -> (w936:string)
                n449 = local write "Report"(w936) -> ()
              }
            }
            n450 = local read "Watchdog config"() -> (w927:T2)
            n451 = Merge Errors(w920, w918) -> (w919:errorcluster)
            n452 = call <vilib>:"Watchdog Configure.vi"("error in (no error)"=w918, "expiration actions"=w927, "timeout (1 sec)"=200.0) -> ("error out"=w928:errorcluster, "watchdogID"=w925:u64)  [unwired: 1 in, 2 out]
            n453 = flat-sequence {
              tunnel: [w946] -> w931
              tunnel: w928 -> [w941]
              tunnel: w919 -> [w959]
              tunnel: [w942] -> w929
              tunnel: w925 -> [w940]
              tunnel: [w939] -> w924
              tunnel: [w938] -> w923
              frame #0 {
                n454 = Get Date/Time In Seconds() -> (seconds since 1Jan1904=w953:timestamp)
                n455 = local read "Ultimo TEST"() -> (w954:timestamp)
                n456 = To Double Precision Float(number=w953) -> (double precision float=w955:dbl)
                n457 = Subtract(x=w955, y=3600.0) -> (x-y=w957:dbl)
                n458 = To Time Stamp(1:w957) -> (0:w958:timestamp)
                n459 = call <vilib>:"Watchdog Whack.vi"("error in (no error)"=w941, "reset watchdog after expire? (F)"=TRUE, "watchdogID in"=w940) -> ("error out"=w938:errorcluster, "watchdogID out"=w939:u64)  [unwired: 2 in, 1 out]
                n460 = In Range and Coerce(upper limit=w953, x=w954, lower limit=w958) -> (In Range?=w952:bool)  [unwired: 1 out]
                n461 = case shown="False" w952 {
                  tunnel: w959 -> [w969 w993]
                  tunnel: [w969 w993] -> w942
                  frame False {
                    n462 = local read "Timeout ruedas"() -> (w970:bool)
                    n463 = local read "Aviso no detección"() -> (w973:string)
                    n464 = local read "Aviso temperatura"() -> (w972:string)
                    n465 = case shown="True" w970 {
                      selector: w970 -> [_ w990]
                      tunnel: ["\r" w991] -> w968
                      frame False {
                      }
                      frame True {
                        w980 = "\n"
                        n466 = local read "Nº Ruedas 1"() -> (w987:i32)
                        n467 = local read "NºRuedas 2"() -> (w982:i32)
                        n468 = call "ErrorRuedas.vi"("Buffer Overflow"=w990) -> ("error out"=w992:errorcluster)
                        n469 = Number To Decimal String(number=w987) -> (decimal integer string=w985:string)  [unwired: 1 in]
                        n470 = Number To Decimal String(number=w982) -> (decimal integer string=w981:string)  [unwired: 1 in]
                        n471 = Concatenate Strings("Error Wheel sensors", "\n", "WS1 (wheels):", w985, w980, "WS2 (wheels):", w981, w980) -> (w983:string)
                        n472 = call "Error.vi"("Error con..."=w983, "error comunicacion 2"=w992) -> ("String"=w991:string)
                      }
                    }
                    n473 = local read "DC OK"() -> (w971:string)
                    n474 = call "Cabecera.vi"() -> ("String"=w978:string)
                    n475 = call "Adquisicion.vi"("Aviso no detección"=w973) -> ("String"=w977:string)
                    n476 = call "Temperatura.vi"("Aviso temperatura"=w972) -> ("String"=w976:string)
                    n477 = call "Fuente.vi"("DC OK"=w971) -> ("String"=w975:string)
                    n478 = call "FPGA.vi"("error out"=w969) -> ("String"=w974:string)
                    n479 = Get Date/Time In Seconds() -> (seconds since 1Jan1904=→"Ultimo TEST":timestamp)
                    n480 = Concatenate Strings(w978, w977, w976, w975, w974, w968) -> (w962:string)
                    n481 = local read "Report"() -> (w961:string)
                    n482 = Concatenate Strings(w962, w961) -> (w963:string)
                    n483 = local read "Max archivos"() -> (w964:u32)
                    n484 = local read "Path LOG"() -> (w967:path)
                    n485 = local read "LOG.txt"() -> (w965:path)
                    n486 = call "Saving_LOG.vi"("Path"=w965, "Report"=w963, "Report AURA"=w962, "Path Carpeta"=w967, "Nº Archivos Max"=w964) -> ("Report"=w966:string)  [unwired: 9 in, 1 out]
                    n487 = local write "Report"(w966) -> ()
                  }
                  frame True {
                  }
                }
                n488 = local read "Fallo fotocelula"() -> (w945:bool)
                n489 = local read "T fuera rango"() -> (w951:bool)
                n490 = Unbundle By Name(w942) -> ("status"=w943:bool)
                n491 = Compound Arithmetic op=OR(w943, w945) -> (w944:bool)
                n492 = local write "Reset del controlador"(w944) -> ()
                n493 = Select(t="UPS", s=w951, f="Espera") -> (s? t:f=w948:string)
                n494 = Select(t="Configuracion", s=w944, f=w948) -> (s? t:f=w946:string)
              }
            }
            n495 = call <vilib>:"Watchdog Clear.vi"("error in (no error)"=w923, "watchdogID in"=w924) -> ("error out"=w921:errorcluster)  [unwired: 5 in]
          }
          frame "Calibracion" {
            n496 = flat-sequence {
              tunnel: w1009 -> [w1789]
              tunnel: w1008 -> [w1788]
              tunnel: [w1789] -> w1007
              tunnel: [w1788] -> w1006
              frame #0 {
                n497 = local read "Report"() -> (w1785:string)
                n498 = call "Reporting_datetime.vi"() -> ("String"=w1784:string)  [unwired: 11 in]
                n499 = Concatenate Strings(w1784, "\nSTATUS: CALIBRATION\n\n\n", w1785) -> (w1787:string)
                n500 = local write "Report"(w1787) -> ()
              }
            }
            n501 = for {
              N: 5 -> [_]
              shift-right: [w1048] -> w1000
              shift-left: w1007 -> [w1050]
              shift-right: [w1047] -> w996
              shift-left: w1006 -> [w1049]
              shift-right: [w1045] -> _
              shift-left: "Adquisicion" ("element") -> [w1046]
              shift-right: [w1044] -> _
              shift-left: _ -> [w1042]
              shift-right: [w1040] -> w995
              shift-left: "" -> [w1039]
              i -> [w1038]
              stop <- w1043 stop-if-true
              n502 = case shown="\"Acel_frequency\"" w1046 {
                tunnel: w1050 -> [w1058 w1288 w1492 w1650 w1735]
                tunnel: w1049 -> [w1057 w1287 w1491 w1649 w1734]
                tunnel: [w1056 w1288 w1492 w1650 w1735] -> w1048
                tunnel: [w1055 w1287 w1491 w1649 w1734] -> w1047
                tunnel: ["Acel_calib" ("Concept") "Acel_frequency" ("Concept") "Acel_noise" ("Concept") "Acel_result" ("Concept") "Adquisicion" ("Concept")] -> w1045
                tunnel: [sgl[][] [] w1284 w1490 w1648 sgl[][] []] -> w1044
                tunnel: [TRUE w1283 w1489 w1645 FALSE] -> w1037
                tunnel: w1042 -> [_ _ w1481 w1651 w1745]
                tunnel: ["\n" w1281 w1487 w1641 w1733] -> w1041
                frame "Adquisicion", Default {
                  n503 = flat-sequence {
                    tunnel: w1057 -> [w1080]
                    tunnel: w1058 -> [w1081]
                    tunnel: [w1081] -> w1061
                    tunnel: [w1080] -> w1060
                    tunnel: [w1064] -> w1059
                    tunnel: w1061 -> [w1093]
                    tunnel: w1060 -> [w1092]
                    tunnel: w1059 -> [w1089]
                    tunnel: [w1091] -> w1056
                    tunnel: [w1090] -> w1055
                    frame #0 {
                      w1076 = "Calibration" ("element")
                      w1075 = "c"
                      n504 = Format Date/Time String(time format string (%c)="%Y-%m-%d-%H-%M-%S") -> (date/time string=w1067:string)  [unwired: 2 in]
                      n505 = for {
                        N: 1 -> [_]
                        shift-right: [w1082] -> w1062
                        shift-left: _ -> [w1083]
                        n506 = Add(x=w1083, y=0.001) -> (x+y=w1082:dbl)
                      }
                      n507 = Number To Fractional String(number=w1062) -> (F-format string=w1071:string)  [unwired: 3 out]
                      n508 = Search and Replace String(input string=w1071, search string="." ("replace string (\"\")")) -> (result string=w1069:string)  [unwired: 1 in, 8 out]
                      n509 = for {
                        N: 3 -> [_]
                        shift-right: [w1087] -> w1065
                        shift-left: w1069 -> [w1085]
                        n510 = Search and Replace String(input string=w1085, search string="0", offset=4 ("offset (0)")) -> (result string=w1087:string)  [unwired: 1 in, 7 out]
                      }
                      n511 = Concatenate Strings(w1065, "_" ("replace string (\"\")"), w1067) -> (w1064:string)
                      "date/time string 2" <- w1064
                      n512 = Build Array(w1075, w1076, w1064) -> (w1074:string[])
                      n513 = Build Array(w1075, w1076, w1064, "Calibration_LOG.txt" ("element")) -> (w1078:string[])
                      n514 = Array of Strings to Path(0:w1074) -> (2:w1073:path)  [unwired: 1 out]
                      "Folder" <- w1073
                      n515 = Array of Strings to Path(0:w1078) -> (2:→"calibration log":path)  [unwired: 1 out]
                      n516 = Create Folder(path (use dialog)=w1073) -> ()  [unwired: 2 in, 3 out]
                    }
                    frame #1 {
                      n517 = for {
                        N: 11 -> [_]
                        shift-right: [w1112] -> w1091
                        shift-left: w1093 -> [w1122]
                        shift-right: [w1115] -> w1090
                        shift-left: w1092 -> [w1121]
                        tunnel: w1089 -> [w1108]
                        i -> [w1118]
                        n518 = xnode "Invoke Method"("FPGA VI Reference In"=w1122, "error in"=w1121) -> ("FPGA VI Reference Out"=w1120:refnum<k20>, "error out"=w1119:errorcluster)  [unwired: 1 in]
                        n519 = Increment(x=w1118) -> (x+1=w1117:i32)
                        n520 = Number To Decimal String(number=w1117) -> (decimal integer string=w1116:string)  [unwired: 1 in]
                        n521 = flat-sequence {
                          tunnel: w1120 -> [w1133]
                          tunnel: w1119 -> [w1132]
                          tunnel: w1116 -> [w1131]
                          tunnel: [w1133] -> w1114
                          tunnel: [w1132] -> w1113
                          tunnel: [w1126] -> w1109
                          tunnel: w1108 -> [w1126]
                          tunnel: [w1125] -> w1095
                          tunnel: w1114 -> [w1141]
                          tunnel: w1113 -> [w1140]
                          tunnel: [w1141] -> w1111
                          tunnel: [w1140] -> w1110
                          tunnel: w1109 -> [w1138]
                          tunnel: [w1138] -> w1107
                          tunnel: [w1137] -> w1096
                          tunnel: w1095 -> [w1137]
                          tunnel: w1111 -> [w1181]
                          tunnel: w1110 -> [w1180]
                          tunnel: w1107 -> [w1159]
                          tunnel: [w1179] -> w1106
                          tunnel: [w1178] -> w1105
                          tunnel: [w1152] -> w1104
                          tunnel: [w1151] -> w1103
                          tunnel: [w1150] -> w1102
                          tunnel: [w1149] -> w1101
                          tunnel: w1096 -> [w1142]
                          tunnel: w1106 -> [w1208]
                          tunnel: w1105 -> [w1209]
                          tunnel: w1104 -> [w1205]
                          tunnel: w1103 -> [w1204]
                          tunnel: w1102 -> [w1203]
                          tunnel: w1101 -> [w1202]
                          tunnel: [w1207] -> w1100
                          tunnel: [w1199] -> w1099
                          tunnel: [w1196] -> w1098
                          tunnel: [w1195] -> w1097
                          tunnel: [w1274] -> w1115
                          tunnel: [w1275] -> w1112
                          tunnel: w1100 -> [w1277]
                          tunnel: w1099 -> [w1276]
                          tunnel: w1098 -> [w1272]
                          tunnel: w1097 -> [w1271]
                          frame #0 {
                            w1123 = dbl[] [] ("mean")
                            n522 = local read "Report"() -> (w1128:string)
                            n523 = local write "mean"(w1123) -> ()
                            n524 = local write "median"(w1123) -> ()
                            n525 = local write "max"(w1123) -> ()
                            n526 = local write "min"(w1123) -> ()
                            n527 = local write "Value to compare"(w1123) -> ()
                            n528 = Concatenate Strings("\nAcquiring file: ", w1131, "/11\n" ("string"), w1128) -> (w1127:string)
                            n529 = for {
                              N: 1 -> [_]
                              shift-right: [w1134] -> w1125
                              shift-left: _ -> [w1135]
                              n530 = Add(x=w1135, y=0.001) -> (x+y=w1134:dbl)
                            }
                            n531 = local write "Report"(w1127) -> ()
                          }
                          frame #1 {
                            n532 = Wait (ms)(milliseconds to wait=u32 1000) -> ()  [unwired: 1 out]
                          }
                          frame #2 {
                            n533 = local read "Frecuencia de muestreo y módulo CRIO"() -> (w1177:T3)
                            n534 = local read "Frecuencia de muestreo (Hz)"() -> (w1175:dbl)
                            n535 = Number To Fractional String(number=w1142) -> (F-format string=w1156:string)  [unwired: 3 out]
                            n536 = local read "Escaneos de la FIFO por canal"() -> (w1174:u32)
                            n537 = xnode "Read/Write Control"("FPGA VI Reference In"=w1181, "error in"=w1180, "Fotocélula"=TRUE ("Adquirir")) -> ("FPGA VI Reference Out"=w1185:refnum<k20>, "error out"=w1184:errorcluster)
                            n538 = local read "Nº de acelerómetros"() -> (w1172:i32)
                            n539 = local read "Count(mSec)"() -> (w1176:u32)
                            n540 = local read "Nº inductivos"() -> (w1173:i32)
                            n541 = Search and Replace String(input string=w1156, search string="." ("replace string (\"\")")) -> (result string=w1154:string)  [unwired: 1 in, 8 out]
                            n542 = for {
                              N: 3 -> [_]
                              shift-right: [w1193] -> w1157
                              shift-left: w1154 -> [w1191]
                              n543 = Search and Replace String(input string=w1191, search string="0", offset=4 ("offset (0)")) -> (result string=w1193:string)  [unwired: 1 in, 7 out]
                            }
                            n544 = xnode "Read/Write Control"("FPGA VI Reference In"=w1185, "error in"=w1184, "Data Rate"=w1177, "Digital?"=TRUE, "Count(mSec)"=w1176) -> ("FPGA VI Reference Out"=w1187:refnum<k20>, "error out"=w1186:errorcluster)
                            n545 = Format Date/Time String(time format string (%c)="%Y-%m-%d-%H-%M-%S") -> (date/time string=w1158:string)  [unwired: 2 in]
                            n546 = Add(x=w1173, y=w1172) -> (x+y=w1171:i32)
                            n547 = call "DMACalc.vi"("Number of Channels"=w1171, "Number of Samples"=w1174, "Rate (Hz)"=w1175) -> ("Block Size"=w1151:u32, "Time to Acquire Block (ms)"=w1152:i32, "Host Buffer Size"=w1170:u32)  [unwired: 6 in]
                            n548 = xnode "Invoke Method"("FPGA VI Reference In"=w1187, "error in"=w1186, "Requested Depth"=w1170) -> ("FPGA VI Reference Out"=w1189:refnum<k20>, "error out"=w1188:errorcluster)  [unwired: 1 out]
                            n549 = Concatenate Strings(w1157, "_" ("replace string (\"\")"), w1158, ".bin" ("string")) -> (w1165:string)
                            n550 = Build Array("c", "Calibration" ("element"), w1159, w1165) -> (w1164:string[])
                            n551 = xnode "Invoke Method"("FPGA VI Reference In"=w1189, "error in"=w1188) -> ("FPGA VI Reference Out"=w1179:refnum<k20>, "error out"=w1178:errorcluster)
                            n552 = local read "Report"() -> (w1144:string)
                            n553 = Array of Strings to Path(0:w1164) -> (2:w1145:path)  [unwired: 1 out]
                            n554 = Path To String(path=w1145) -> (string=w1148:string)
                            n555 = Get Date/Time In Seconds() -> (seconds since 1Jan1904=→"Inicio pasada 2":timestamp)
                            n556 = Concatenate Strings("\nFile created: ", w1148, "\n", w1144) -> (w1143:string)
                            n557 = Open/Create/Replace File(file path (use dialog)=w1145, operation (0:open)=T5."replace or create", access (0:read/write)=enum16{"read/write", "read-only", "write-only"}."read/write", disable buffering (F)=TRUE) -> (refnum out=w1150:refnum<file>, error out=w1149:errorcluster)  [unwired: 1 in, 2 out]
                            n558 = local write "Report"(w1143) -> ()
                          }
                          frame #3 {
                            n559 = while "Data Acquisition" {
                              tunnel: w1208 -> [w1234]
                              shift-right: [w1241] -> _
                              shift-left: u32 0 ("t") -> [w1237]
                              tunnel: w1205 -> [w1242]
                              tunnel: w1204 -> [w1240]
                              shift-right: [w1243] -> w1199
                              shift-left: w1209 -> [w1233]
                              tunnel: [w1238] -> w1207
                              tunnel: w1203 -> [w1223]
                              tunnel: [w1224] -> w1196
                              shift-right: [w1222] -> w1195
                              shift-left: w1202 -> [w1231]
                              stop <- w1239 stop-if-true
                              # "Detector de presencia"
                              # "Mide el tiempo de paso del tren y con ello se puede calcular\nla velocidad la unidad"
                              n560 = xnode "Invoke Method"("FPGA VI Reference In"=w1234, "error in"=w1233, "Number of Elements"=w1237, "Timeout (ms)"=0) -> ("FPGA VI Reference Out"=w1221:refnum<k20>, "error out"=w1220:errorcluster, "Data"=w1232:fxp<+/-,24,4>[], "Elements Remaining"=w1235:u32)
                              n561 = case "Data Ready" shown="Default" w1237 {
                                tunnel: w1242 -> [w1248 _]
                                tunnel: [w1247 u32 0 ("t")] -> w1241
                                tunnel: w1240 -> [w1249 _]
                                tunnel: w1235 -> [w1246 _]
                                tunnel: w1232 -> [_ w1259]
                                tunnel: w1231 -> [w1245 w1261]
                                tunnel: [w1245 w1260] -> w1222
                                tunnel: w1223 -> [w1244 w1258]
                                tunnel: [w1244 w1257] -> w1224
                                frame 0 {
                                n562 = Greater Or Equal?(x=w1246, y=w1249) -> (x >= y?=w1250:bool)
                                n563 = case shown="False" w1250 {
                                tunnel: [u32 0 ("Block Size") w1254] -> w1247
                                tunnel: [w1253 0 ("t")] -> w1251
                                tunnel: w1248 -> [w1253 _]
                                tunnel: w1249 -> [_ w1254]
                                frame False {
                                }
                                frame True {
                                }
                                }
                                n564 = call "WaitMinTimeBetweenCall.vi"("Minimum ms between calls"=w1251) -> ()  [unwired: 2 in]
                                }
                                frame Default {
                                n565 = To Single Precision Float(number=w1259) -> (single precision float=w1256:sgl[])
                                n566 = Write to Binary File(file (use dialog)=w1258, data=w1256, error in=w1261, 5:FALSE ("prepend array or string size? (T)"), 9:T6."little-endian" ("byte order (0:big-endian, network order)")) -> (refnum out=w1257:refnum<file>, error out=w1260:errorcluster)  [unwired: 2 out]
                                }
                              }
                              n567 = local read "Inicio pasada 2"() -> (w1212:timestamp)
                              n568 = Get Date/Time In Seconds() -> (seconds since 1Jan1904=w1213:timestamp)
                              n569 = xnode ("CheckLate")("FPGA VI Reference In"=w1221, "error in"=w1220) -> ("FPGA VI Reference Out"=w1215:refnum<k20>, "error out"=w1229:errorcluster, "Buffer Underflow"=w1210:bool, "Buffer Overflow"=w1211:bool)
                              n570 = To Double Precision Float(number=w1213) -> (double precision float=w1218:dbl)
                              n571 = To Double Precision Float(number=w1212) -> (double precision float=w1219:dbl)
                              n572 = Subtract(x=w1218, y=w1219) -> (x-y=w1226:dbl)
                              "Acquiring time" <- w1226
                              n573 = local write "Buffer Overflow"(w1211) -> ()
                              n574 = local write "Buffer Underflow"(w1210) -> ()
                              n575 = Greater?(x=w1226, y=1.0 ("Tiempo de adquisición")) -> (0:w1217:bool)
                              n576 = call "ErrorOverFlow.vi"("Buffer Overflow"=w1211) -> ("error out"=w1227:errorcluster)
                              n577 = call "ErrorUnderFlow.vi"("Buffer Overflow"=w1210) -> ("error out"=w1228:errorcluster)
                              n578 = Merge Errors(w1229, w1228, w1227) -> (w1216:errorcluster)
                              n579 = Unbundle By Name(w1222) -> ("status"=w1225:bool)
                              n580 = Unbundle By Name(w1216) -> ("status"=w1230:bool)
                              n581 = Compound Arithmetic op=OR(w1230, w1217, w1225) -> (w1239:bool)
                              n582 = case "Flush" shown="True" w1239 {
                                tunnel: w1215 -> [w1265 w1270]
                                tunnel: w1216 -> [w1266 w1269]
                                tunnel: [w1266 w1268] -> w1243
                                tunnel: [w1265 w1267] -> w1238
                                frame False {
                                }
                                frame True {
                                n583 = xnode "Invoke Method"("FPGA VI Reference In"=w1270, "error in"=w1269) -> ("FPGA VI Reference Out"=w1267:refnum<k20>, "error out"=w1268:errorcluster)
                                }
                              }
                            }
                            n584 = call "Reporting_error.vi"("error out 2"=w1199, "Concept"="FPGA ") -> ("Reporting"=w1201:string)  [unwired: 1 in]
                            n585 = local read "Report"() -> (w1198:string)
                            n586 = Concatenate Strings(w1201, w1198) -> (w1200:string)
                            n587 = local write "Report"(w1200) -> ()
                          }
                          frame #4 {
                            n588 = xnode "Read/Write Control"("FPGA VI Reference In"=w1277, "error in"=w1276, "Stop"=TRUE) -> ("FPGA VI Reference Out"=w1278:refnum<k20>, "error out"=w1279:errorcluster)
                            n589 = Close File(refnum=w1272, error in=w1271) -> ()  [unwired: 2 out]
                            n590 = xnode "Invoke Method"("FPGA VI Reference In"=w1278, "error in"=w1279) -> ("FPGA VI Reference Out"=w1275:refnum<k20>, "error out"=w1274:errorcluster)
                          }
                        }
                      }
                    }
                  }
                }
                frame "Acel_calib" {
                  n591 = local read "Folder"() -> (w1290:path)
                  n592 = local read "Frecuencia de muestreo (Hz)"() -> (w1296:dbl)
                  n593 = local read "Nº de acelerómetros"() -> (w1291:i32)
                  n594 = local read "Nº inductivos"() -> (w1292:i32)
                  n595 = local read "Pattern frequency (Hz)"() -> (w1297:dbl)
                  n596 = call <vilib>:"Recursive File List.vi"("Folder Path"=w1290) -> ("All Files in Dir"=w1295:path[])  [unwired: 6 in, 4 out]
                  n597 = Array Size(array=w1295) -> (size(s)=→"Nº meas":i32)
                  n598 = Add(x=w1292, y=w1291) -> (x+y=w1294:i32)
                  n599 = flat-sequence {
                    tunnel: w1295 -> [w1307]
                    tunnel: [w1307] -> w1303
                    tunnel: [w1306] -> w1302
                    tunnel: w1294 -> [w1306]
                    tunnel: [w1305] -> w1301
                    tunnel: w1296 -> [w1305]
                    tunnel: [w1304] -> w1300
                    tunnel: w1297 -> [w1304]
                    tunnel: [w1314] -> w1299
                    tunnel: [w1313] -> w1298
                    tunnel: w1303 -> [w1315]
                    tunnel: w1302 -> [w1312]
                    tunnel: w1301 -> [w1311]
                    tunnel: w1300 -> [w1310]
                    tunnel: [w1309] -> w1280
                    tunnel: w1299 -> [w1427]
                    tunnel: w1298 -> [w1416]
                    tunnel: [w1408] -> w1284
                    tunnel: [TRUE] -> w1283
                    tunnel: [w1442] -> w1281
                    tunnel: [w1417] -> w1282
                    tunnel: w1280 -> [w1412]
                    frame #0 {
                      "Valid\nindex" <- i32[] []
                    }
                    frame #1 {
                      n600 = for {
                        tunnel: w1315 -> [w1337] mode=indexing
                        tunnel: [w1327] -> w1314 mode=indexing
                        tunnel: [w1317] -> w1313 mode=indexing
                        tunnel: w1312 -> [w1325]
                        tunnel: w1311 -> [w1324]
                        tunnel: w1310 -> [w1323]
                        tunnel: [w1316] -> w1309 mode=indexing
                        n601 = Read from Binary File(5:sgl 1.25, 9:T6."little-endian" ("byte order (0:big-endian, network order)"), 10:-1 ("count (1)"), 11:w1337) -> (2:w1338:sgl[])  [unwired: 1 in, 4 out]
                        n602 = case shown="10" w1325 {
                          tunnel: [w1355 w1368 w1378] -> w1317
                          tunnel: w1338 -> [w1356 w1366 w1379]
                          frame 9, Default {
                            n603 = Decimate 1D Array(w1356) -> (w1357:sgl[], w1365:sgl[], w1364:sgl[], w1360:sgl[], w1359:sgl[], w1361:sgl[], w1362:sgl[], w1363:sgl[], w1358:sgl[])
                            n604 = Build Array(w1357, w1365, w1364, w1360, w1359, w1361, w1362, w1363, w1358) -> (w1355:sgl[][])
                          }
                          frame 10 {
                            n605 = Decimate 1D Array(w1366) -> (w1367:sgl[], w1377:sgl[], w1376:sgl[], w1372:sgl[], w1371:sgl[], w1373:sgl[], w1374:sgl[], w1375:sgl[], w1370:sgl[], w1369:sgl[])
                            n606 = Build Array(w1367, w1377, w1376, w1372, w1371, w1373, w1374, w1375, w1370, w1369) -> (w1368:sgl[][])
                          }
                          frame 5 {
                            n607 = Decimate 1D Array(w1379) -> (w1380:sgl[], w1384:sgl[], w1383:sgl[], w1382:sgl[], w1381:sgl[])
                            n608 = Build Array(w1380, w1384, w1383, w1382, w1381) -> (w1378:sgl[][])
                          }
                        }
                        n609 = for {
                          tunnel: w1317 -> [w1387] mode=indexing
                          tunnel: [w1390] -> w1334 mode=indexing
                          tunnel: w1324 -> [w1389]
                          tunnel: w1323 -> [w1388]
                          n610 = call-poly <vilib>:"Basic Averaged DC-RMS.vi"("signal in"=w1387) -> ("DC value"=w1400:dbl)  [unwired: 7 in, 3 out]
                          n611 = Array Size(array=w1387) -> (size(s)=→"size(s) 3":i32)
                          n612 = Subtract(x=w1387, y=w1400) -> (x-y=w1396:dbl[])
                          n613 = Divide(x=w1389, y=w1388) -> (x/y=w1397:dbl)
                          n614 = Array Size(array=w1396) -> (size(s)=w1398:i32)
                          n615 = Subtract(x=w1398, y=w1397) -> (x-y=w1399:dbl)
                          n616 = for {
                            N: w1399 -> [_]
                            tunnel: w1397 -> [w1402]
                            tunnel: [w1405] -> w1385 mode=indexing
                            tunnel: w1396 -> [w1404]
                            i -> [w1403]
                            n617 = Array Subset(array=w1404, index=w1403, length=w1402) -> (w1401:dbl[])
                            n618 = call-poly <vilib>:"RMS.vi"("X"=w1401) -> ("rms value"=w1405:dbl)  [unwired: 1 out]
                          }
                          n619 = Greater?(x=w1385, y=0.004 ("threshold y")) -> (0:w1394:bool[])
                          n620 = Search 1D Array(1D array=w1394, element=TRUE) -> (index of element=w1392:i32)  [unwired: 1 in]
                          n621 = Not Equal?(x=w1392, y=-1) -> (x != y?=w1390:bool)
                        }
                        n622 = Array Size(array=w1317) -> (size(s)=→"size(s)":i32[])
                        n623 = while {
                          tunnel: w1334 -> [w1354]
                          shift-right: [w1346] -> _
                          shift-left: 0 ("index of element") -> [w1351]
                          shift-right: [w1347] -> w1326
                          shift-left: 0 ("index of element") -> [w1348]
                          tunnel: [w1345] -> w1322 mode=indexing
                          i -> [w1349]
                          stop <- w1352 stop-if-true
                          n624 = Add(x=w1348, y=w1349) -> (x+y=w1347:i32)
                          n625 = Search 1D Array(1D array=w1354, element=TRUE, start index (0)=w1351) -> (index of element=w1345:i32)
                          n626 = Equal?(x=w1345, y=-1) -> (x = y?=w1352:bool)
                          n627 = Increment(x=w1345) -> (x+1=w1346:i32)
                        }
                        n628 = Delete From Array(array=w1322, length=1) -> (array with subset deleted=w1321:i32[])  [unwired: 1 in, 1 out]
                        n629 = Array Size(array=w1321) -> (size(s)=w1330:i32)
                        n630 = Equal?(x=w1326, y=1) -> (x = y?=w1329:bool)
                        n631 = Equal?(x=w1330, y=1) -> (x = y?=w1328:bool)
                        n632 = And(x=w1328, y=w1329) -> (x .and. y?=w1327:bool)
                        n633 = case shown="True" w1327 {
                          tunnel: w1321 -> [_ w1344]
                          frame False {
                          }
                          frame True {
                            n634 = local read "Valid\nindex"() -> (w1342:i32[])
                            n635 = Insert Into Array(array=w1342, new element=w1344) -> (w1343:i32[])  [unwired: 1 in]
                            n636 = local write "Valid\nindex"(w1343) -> ()
                          }
                        }
                        n637 = Array Size(array=w1317) -> (size(s)=w1319:i32[])
                        n638 = Index Array(array=w1319, index=1) -> (element=w1316:i32)
                      }
                    }
                    frame #2 {
                      w1426 = 0 ("index of element")
                      (unwired) 0 ("index of element")
                      n639 = local read "Valid\nindex"() -> (w1432:i32[])
                      n640 = Array Max & Min(array=w1412) -> (min value=w1409:i32)  [unwired: 3 out]
                      n641 = Sort 1D Array(array=w1432) -> (sorted array=w1428:i32[])
                      "sorted array" <- w1428
                      n642 = Decrement(x="Accelerometer") -> (x-1=w1407:i32)
                      n643 = for {
                        tunnel: w1428 -> [w1463] mode=indexing
                        shift-right: [w1463] -> _
                        shift-left: -1 ("y") -> [w1464]
                        tunnel: [w1463] -> w1437 mode=indexing if=w1462
                        shift-right: [w1459] -> _
                        shift-left: 0 ("y") -> [w1460]
                        tunnel: [w1459] -> w1435 mode=indexing
                        n644 = Not Equal?(x=w1463, y=w1464) -> (x != y?=w1462:bool)
                        n645 = Increment(x=w1460) -> (x+1=w1461:i32)
                        n646 = Select(t=1 ("y"), s=w1462, f=w1461) -> (s? t:f=w1459:i32)
                      }
                      "Array" <- w1437
                      "Array 3" <- w1435
                      n647 = Delete From Array(array=w1416, index (dim 1)=w1407) -> (deleted portion=w1410:sgl[][])  [unwired: 3 in, 1 out]
                      n648 = for {
                        tunnel: w1427 -> [w1469] mode=indexing
                        shift-right: [w1468] -> _
                        shift-left: w1416 -> [w1470]
                        shift-right: [w1465] -> _
                        shift-left: 0 ("index of element") -> [w1466]
                        i -> [w1467]
                        n649 = case shown="False" w1469 {
                          tunnel: w1470 -> [w1476 w1478]
                          tunnel: [w1475 w1478] -> w1468
                          tunnel: w1467 -> [w1474 _]
                          tunnel: w1466 -> [w1471 w1477]
                          tunnel: [w1472 w1477] -> w1465
                          frame False {
                            n650 = Subtract(x=w1474, y=w1471) -> (x-y=w1473:i32)
                            n651 = Delete From Array(array=w1476, index (dim 0)=w1473) -> (array with subset deleted=w1475:sgl[][][])  [unwired: 3 in, 1 out]
                            n652 = Increment(x=w1471) -> (x+1=w1472:i32)
                          }
                          frame True {
                          }
                        }
                      }
                      n653 = Array Subset(array=w1410, index (col)=0 ("index"), length (col)=w1409) -> (w1408:sgl[][])  [unwired: 2 in]
                      n654 = Array Max & Min(array=w1435) -> (max value=→"max value":i32, max index (indices)=w1433:i32)  [unwired: 2 out]
                      "max index(es)" <- w1433
                      n655 = Index Array(array=w1428, index=w1433) -> (element=w1417:i32)
                      "element" <- w1417
                      n656 = local read "Frecuencia de muestreo (Hz)"() -> (w1415:dbl)
                      n657 = Equal?(x=w1432, y=w1417) -> (x = y?=w1430:bool[])
                      n658 = Boolean To (0,1)(Boolean=w1430) -> (0, 1=w1429:i16[])
                      n659 = Add Array Elements(numeric array=w1429) -> (sum=w1421:i16)
                      n660 = Equal?(x=w1417, y=w1426) -> (x = y?=w1424:bool)
                      n661 = Equal?(x=w1426, y=w1421) -> (x = y?=w1423:bool)
                      n662 = Increment(x=w1417) -> (x+1=w1431:i32)
                      n663 = local read "Nº meas"() -> (w1443:i32)
                      n664 = Not And(1:w1423, 2:w1424) -> (0:w1422:bool)
                      n665 = for {
                        tunnel: w1408 -> [w1457] mode=indexing
                        tunnel: w1415 -> [w1455]
                        tunnel: [w1454] -> w1414 mode=indexing
                        n666 = Reciprocal(x=w1455) -> (1/x=w1456:dbl)
                        n667 = Bundle By Name("Y"=w1457, "dt"=w1456) -> (w1454:waveform(sgl))  [unwired: 1 in]
                      }
                      n668 = Number To Decimal String(number=w1431) -> (decimal integer string=w1419:string)  [unwired: 1 in]
                      n669 = Select(t=w1419, s=w1422, f=" NONE ") -> (s? t:f=w1420:string)
                      n670 = Number To Decimal String(number=w1421) -> (decimal integer string=w1449:string)  [unwired: 1 in]
                      n671 = Number To Decimal String(number=w1443) -> (decimal integer string=w1447:string)  [unwired: 1 in]
                      n672 = Divide(x=w1421, y=w1443) -> (x/y=w1445:dbl)
                      n673 = for {
                        tunnel: w1414 -> [w1453] mode=indexing
                        tunnel: [w1450] -> w1413 mode=concatenating
                        n674 = call "Convert to Dynamic Data"("Waveform"=w1453) -> ("Dynamic Data Type"=w1452:dynamicdata)  [unwired: 3 in]
                        n675 = call "Tone Measurements"("Signals"=w1452) -> ("Frequency"=w1451:dynamicdata)  [unwired: 9 in, 1 out]
                        n676 = call "Convert from Dynamic Data"("Dynamic Data Type"=w1451) -> ("Array"=w1450:dbl[])  [unwired: 3 in]
                      }
                      "Frequency" <- w1413
                      n677 = Greater?(x=w1445, y=0.6) -> ()  [unwired: 1 out]
                      n678 = Concatenate Strings("\nACCELEROMETER DETECTOR:\n\nAccelerometer detected: ", w1420, " \nAccelerometer detected in  ", w1449, " of ", w1447, " measurements\n------------------------------------------------------------------------------------------------------------------------------------------------") -> (w1442:string)
                    }
                  }
                  n679 = local read "Report"() -> (w1285:string)
                  n680 = Concatenate Strings(w1281, w1285) -> (w1286:string)
                  n681 = local write "Report"(w1286) -> ()
                  "Accel.detected" <- w1282
                }
                frame "Acel_frequency" {
                  n682 = local read "Low cutoff freq"() -> (w1483:dbl)
                  n683 = local read "Frequency"() -> (w1484:dbl[])
                  n684 = local read "Frecuencia de muestreo (Hz)"() -> (w1485:dbl)
                  n685 = local read "Pattern frequency (Hz)"() -> (w1486:dbl)
                  n686 = Less?(x=w1484, y=w1483) -> (x < y?=w1479:bool[])
                  n687 = for {
                    tunnel: w1479 -> [w1503] mode=indexing
                    shift-right: [w1502] -> w1480
                    shift-left: w1481 -> [w1504]
                    shift-right: [w1499] -> _
                    shift-left: 0 ("index of element") -> [w1500]
                    i -> [w1501]
                    n688 = case shown="False" w1503 {
                      tunnel: w1504 -> [w1510 w1512]
                      tunnel: [w1509 w1512] -> w1502
                      tunnel: w1501 -> [w1508 _]
                      tunnel: w1500 -> [w1505 w1511]
                      tunnel: [w1506 w1511] -> w1499
                      frame False {
                        n689 = Subtract(x=w1508, y=w1505) -> (x-y=w1507:i32)
                        n690 = Delete From Array(array=w1510, index (row)=w1507) -> (array with subset deleted=w1509:sgl[][])  [unwired: 2 in, 1 out]
                        n691 = Increment(x=w1505) -> (x+1=w1506:i32)
                      }
                      frame True {
                      }
                    }
                  }
                  n692 = flat-sequence {
                    tunnel: w1480 -> [w1519]
                    tunnel: w1485 -> [w1516]
                    tunnel: w1486 -> [w1513]
                    tunnel: [w1521] -> w1498
                    tunnel: [w1515] -> w1497
                    tunnel: [w1514] -> w1496
                    tunnel: [w1513] -> w1495
                    tunnel: w1498 -> [w1598]
                    tunnel: w1497 -> [w1580]
                    tunnel: w1496 -> [w1597]
                    tunnel: w1495 -> [w1596]
                    tunnel: [w1598] -> w1490
                    tunnel: [w1582] -> w1487
                    tunnel: [w1581] -> w1489
                    tunnel: [w1580] -> _
                    frame #0 {
                      n693 = for {
                        tunnel: w1519 -> [w1571] mode=indexing
                        tunnel: w1516 -> [w1570]
                        tunnel: w1513 -> [w1566]
                        tunnel: [w1547] -> w1515 mode=indexing
                        tunnel: [w1541] -> w1514 mode=indexing
                        n694 = Reciprocal(x=w1570) -> (1/x=w1572:dbl)
                        n695 = Bundle By Name("Y"=w1571, "dt"=w1572) -> (w1569:waveform(sgl))  [unwired: 1 in]
                        n696 = call-poly <vilib>:"FFT Spectrum (Mag-Phase).vi"("time signal"=w1569) -> ("magnitude"=w1568:cluster{"f0":dbl, "df":dbl, "magnitude":dbl[]})  [unwired: 6 in, 4 out]
                        n697 = Unbundle By Name(w1568) -> ("magnitude"=w1560:dbl[], "df"=w1542:dbl)
                        n698 = Multiply(x=1.03, y=w1566) -> (x*y=w1563:dbl)
                        n699 = Multiply(x=w1566, y=0.97 ("x")) -> (x*y=w1564:dbl)
                        n700 = Divide(x=w1564, y=w1542) -> (x/y=w1561:dbl)
                        n701 = Divide(x=w1563, y=w1542) -> (x/y=w1558:dbl)
                        n702 = Array Max & Min(array=w1560) -> (max value=w1553:dbl, max index (indices)=w1543:i32)  [unwired: 2 out]
                        n703 = Array Size(array=w1560) -> (size(s)=w1559:i32)
                        n704 = Multiply(x=w1543, y=w1542) -> (x*y=w1541:dbl)
                        n705 = Subtract(x=w1559, y=w1558) -> (x-y=w1557:dbl)
                        n706 = In Range and Coerce(upper limit=w1563, x=w1541, lower limit=w1564) -> (In Range?=w1546:bool)  [unwired: 1 out]
                        n707 = Array Subset(array=w1560, index=w1558, length=w1557) -> (w1556:dbl[])
                        n708 = Array Subset(array=w1560, index=0, length=w1561) -> (w1555:dbl[])
                        n709 = Array Max & Min(array=w1556) -> (max value=w1554:dbl)  [unwired: 3 out]
                        n710 = Array Max & Min(array=w1555) -> (max value=w1552:dbl)  [unwired: 3 out]
                        n711 = Divide(x=w1553, y=w1552) -> (x/y=w1550:dbl)
                        n712 = Divide(x=w1553, y=w1554) -> (x/y=w1551:dbl)
                        n713 = Greater?(x=w1551, y=3.0) -> (0:w1545:bool)
                        n714 = Greater?(x=w1550, y=3.0) -> (0:w1544:bool)
                        n715 = Compound Arithmetic op=AND(w1546, w1545, w1544) -> (w1547:bool)
                      }
                      n716 = for {
                        shift-right: [w1528] -> w1521
                        shift-left: w1519 -> [w1529]
                        tunnel: w1515 -> [w1527] mode=indexing
                        shift-right: [w1524] -> _
                        shift-left: 0 ("index of element") -> [w1525]
                        shift-right: [w1522] -> w1518
                        shift-left: w1514 -> [w1523]
                        i -> [w1526]
                        n717 = case shown="True" w1527 {
                          tunnel: w1529 -> [w1537 w1540]
                          tunnel: [w1536 w1540] -> w1528
                          tunnel: w1526 -> [w1535 _]
                          tunnel: w1525 -> [w1534 w1539]
                          tunnel: [w1533 w1539] -> w1524
                          tunnel: w1523 -> [w1532 w1538]
                          tunnel: [w1530 w1538] -> w1522
                          frame False {
                            n718 = Subtract(x=w1535, y=w1534) -> (x-y=w1531:i32)
                            n719 = Delete From Array(array=w1537, index (row)=w1531) -> (array with subset deleted=w1536:sgl[][])  [unwired: 2 in, 1 out]
                            n720 = Increment(x=w1534) -> (x+1=w1533:i32)
                            n721 = Delete From Array(array=w1532, index=w1531) -> (array with subset deleted=w1530:dbl[])  [unwired: 1 in, 1 out]
                          }
                          frame True {
                          }
                        }
                      }
                      n722 = call <vilib>:"Std Deviation and Variance.vi"("X"=w1518) -> ("mean"=→"Mean\nfrequency":dbl)  [unwired: 1 in, 2 out]
                    }
                    frame #1 {
                      w1577 = "\r"
                      n723 = for {
                        tunnel: w1580 -> [w1606] mode=indexing
                        tunnel: w1597 -> [w1625] mode=indexing
                        tunnel: w1596 -> [w1624]
                        tunnel: [w1607] -> w1594 mode=indexing
                        shift-right: [w1601] -> w1592
                        shift-left: 0 -> [w1602]
                        i -> [w1627]
                        n724 = Increment(x=w1627) -> (x+1=w1626:i32)
                        n725 = Select(t=1, s=w1606, f=0) -> (s? t:f=w1603:i32)
                        n726 = Divide(x=w1625, y=w1624) -> (x/y=w1622:dbl)
                        n727 = Select(t="TRUE", s=w1606, f="FALSE") -> (s? t:f=w1616:string)
                        n728 = Number To Decimal String(number=w1626) -> (decimal integer string=w1619:string)  [unwired: 1 in]
                        n729 = Number To Fractional String(number=w1625, precision (6)=i16 2) -> (F-format string=w1613:string)  [unwired: 2 in]
                        n730 = Add(x=w1603, y=w1602) -> (x+y=w1601:i32)
                        n731 = Greater Than 0?(x=w1622) -> (x > 0?=w1623:bool)
                        n732 = case shown="True" w1623 {
                          tunnel: w1622 -> [w1635 w1637]
                          tunnel: [w1631 w1639] -> w1621
                          tunnel: ["-" " "] -> w1611
                          frame False {
                            n733 = Subtract(x=1.0, y=w1635) -> (x-y=w1633:dbl)
                            n734 = Multiply(x=100.0, y=w1633) -> (x*y=w1631:dbl)
                          }
                          frame True {
                            n735 = Decrement(x=w1637) -> (x-1=w1638:dbl)
                            n736 = Multiply(x=100.0, y=w1638) -> (x*y=w1639:dbl)
                          }
                        }
                        n737 = Number To Fractional String(number=w1621, precision (6)=i16 2) -> (F-format string=w1610:string)  [unwired: 2 in]
                        n738 = Concatenate Strings("\n\nMeasurement: ", w1619, "\r", "Frequency valid: ", w1616, "\r", "Frequency: ", w1613, ", ", w1611, w1610, " % of error in frequency", "\r") -> (w1607:string)
                      }
                      n739 = Array Size(array=w1580) -> (size(s)=w1591:i32)
                      n740 = Number To Decimal String(number=w1591) -> (decimal integer string=w1586:string)  [unwired: 1 in]
                      n741 = Number To Decimal String(number=w1592) -> (decimal integer string=w1578:string)  [unwired: 1 in]
                      n742 = Divide(x=w1592, y=w1591) -> (x/y=w1575:dbl)
                      n743 = Greater?(x=w1575, y=0.8) -> (0:w1581:bool)
                      n744 = Multiply(x=100.0, y=w1575) -> (x*y=w1574:dbl)
                      n745 = Number To Fractional String(number=w1574, precision (6)=i16 2) -> (F-format string=w1585:string)  [unwired: 2 in]
                      n746 = Select(t="OK\n------------------------------------------------------------------------", s=w1581, f="FAIL (REPEAT ACEL CALIBRATION)\n------------------------------------------------------------------------") -> (s? t:f=w1583:string)
                      n747 = Concatenate Strings("FREQUENCY TEST:\n \n- MEASUREMENT OK IF +/- 5% FREQ PATTERN\n\n- FREQUENCY ANALYSYS MORE THAN 80% OF THE MEASUREMENTS INSIDE OF THE RANGE\n", w1594, w1577, w1577, w1578, " measurements OK of ", w1586, " , ", w1585, " %\n\nFREQUENCY ANALYSIS: ", w1583) -> (w1582:string)
                    }
                  }
                  n748 = local read "Report"() -> (w1494:string)
                  n749 = Concatenate Strings(w1487, w1494) -> (w1493:string)
                  n750 = local write "Report"(w1493) -> ()
                }
                frame "Acel_noise" {
                  n751 = local read "Frecuencia de muestreo (Hz)"() -> (w1644:dbl)
                  n752 = local read "Pattern frequency (Hz)"() -> (w1643:dbl)
                  n753 = flat-sequence {
                    tunnel: w1651 -> [w1662]
                    tunnel: [w1678] -> w1648
                    tunnel: w1644 -> [w1677]
                    tunnel: w1643 -> [w1676]
                    tunnel: [w1665] -> w1641
                    tunnel: [w1664] -> w1645
                    frame #0 {
                      n754 = for {
                        tunnel: w1662 -> [w1726] mode=indexing
                        tunnel: [w1719] -> w1682 mode=indexing
                        tunnel: w1677 -> [w1714]
                        tunnel: w1676 -> [w1715]
                        n755 = call-poly <vilib>:"Basic Averaged DC-RMS.vi"("signal in"=w1726) -> ("DC value"=w1727:dbl)  [unwired: 7 in, 3 out]
                        n756 = Subtract(x=w1726, y=w1727) -> (x-y=w1716:dbl[])
                        n757 = Divide(x=w1714, y=w1715) -> (x/y=w1723:dbl)
                        n758 = Array Size(array=w1716) -> (size(s)=w1724:i32)
                        n759 = Subtract(x=w1724, y=w1723) -> (x-y=w1725:dbl)
                        n760 = for {
                          N: w1725 -> [_]
                          tunnel: w1723 -> [w1729]
                          tunnel: [w1732] -> w1717 mode=indexing
                          tunnel: w1716 -> [w1731]
                          i -> [w1730]
                          n761 = Array Subset(array=w1731, index=w1730, length=w1729) -> (w1728:dbl[])
                          n762 = call-poly <vilib>:"RMS.vi"("X"=w1728) -> ("rms value"=w1732:dbl)  [unwired: 1 out]
                        }
                        n763 = Array Max & Min(array=w1717) -> (max value=w1721:dbl, min value=w1720:dbl)  [unwired: 2 out]
                        n764 = call <vilib>:"Std Deviation and Variance.vi"("X"=w1717) -> ("mean"=w1718:dbl)  [unwired: 1 in, 2 out]
                        n765 = call <vilib>:"Median.vi"("X"=w1717) -> ("median"=w1722:dbl)  [unwired: 1 out]
                        n766 = Build Array(w1718, w1722, w1721, w1720) -> (w1719:dbl[])
                      }
                      n767 = Multiply(x=w1682, y=1000 ("median")) -> (x*y=w1661:dbl[][])
                      n768 = Index Array(array=w1661, index (col) #1=0 ("disabled index (col)"), index (col) #2=1 ("index (col)"), index (col) #3=2 ("index (col)"), index (col) #4=3 ("index (col)")) -> (element #1=→"mean":dbl[], element #2=→"median":dbl[], element #3=→"max":dbl[], element #4=→"min":dbl[])  [unwired: 4 in]
                      n769 = for {
                        tunnel: w1661 -> [w1709] mode=indexing
                        tunnel: [w1706] -> w1663 mode=indexing
                        tunnel: [w1704] -> w1652 mode=indexing
                        (unwired) 0.2 ("x")
                        n770 = local read "noise_range"() -> (w1705:dbl)
                        n771 = call <vilib>:"Median.vi"("X"=w1709) -> ("median"=w1704:dbl)  [unwired: 1 out]
                        n772 = Subtract(x=w1704, y=w1705) -> (x-y=w1707:dbl)
                        n773 = Add(x=w1705, y=w1704) -> (x+y=w1708:dbl)
                        n774 = for {
                          tunnel: w1709 -> [w1713] mode=indexing
                          tunnel: w1708 -> [w1712]
                          tunnel: w1707 -> [w1711]
                          tunnel: [w1710] -> w1706 mode=indexing
                          n775 = In Range and Coerce(upper limit=w1712, x=w1713, lower limit=w1711) -> (In Range?=w1710:bool)  [unwired: 1 out]
                        }
                      }
                      "Value to compare" <- w1652
                      n776 = for {
                        tunnel: w1663 -> [w1703] mode=indexing
                        tunnel: [w1702] -> w1679 mode=indexing
                        n777 = And Array Elements(Boolean array=w1703) -> (logical AND=w1702:bool)
                      }
                      n778 = for {
                        shift-right: [w1689] -> w1678
                        shift-left: w1662 -> [w1690]
                        tunnel: w1679 -> [w1688] mode=indexing
                        shift-right: [w1685] -> w1675
                        shift-left: 0 ("index of element") -> [w1686]
                        shift-right: [w1683] -> w1670
                        shift-left: 0 ("index of element") -> [w1684]
                        i -> [w1687]
                        n779 = case shown="False" w1688 {
                          tunnel: w1690 -> [w1697 w1701]
                          tunnel: [w1696 w1701] -> w1689
                          tunnel: w1687 -> [w1695 _]
                          tunnel: w1686 -> [w1694 w1700]
                          tunnel: [w1693 w1700] -> w1685
                          tunnel: w1684 -> [w1691 w1699]
                          tunnel: [w1691 w1698] -> w1683
                          frame False {
                            n780 = Subtract(x=w1695, y=w1694) -> (x-y=w1692:i32)
                            n781 = Delete From Array(array=w1697, index (row)=w1692) -> (array with subset deleted=w1696:sgl[][])  [unwired: 2 in, 1 out]
                            n782 = Increment(x=w1694) -> (x+1=w1693:i32)
                          }
                          frame True {
                            n783 = Increment(x=w1699) -> (x+1=w1698:i32)
                          }
                        }
                      }
                      n784 = Number To Decimal String(number=w1675) -> (decimal integer string=w1673:string)  [unwired: 1 in]
                      n785 = Greater?(x=w1670, y=3) -> (0:w1664:bool)
                      n786 = Select(t="------------------------------------------------------------------------", s=w1664, f="There are not enough correct measurements to calibrate\n\nREPEAT THE ACCELEROMETER CALIBRATION\n------------------------------------------------------------------------") -> (s? t:f=w1666:string)
                      n787 = Concatenate Strings("SIGNAL NOISE ANALYSIS:\n\nFiles erasing by  noise: ", w1673, "\r", w1666) -> (w1665:string)
                    }
                  }
                  n788 = local read "Report"() -> (w1646:string)
                  n789 = Concatenate Strings(w1641, w1646) -> (w1647:string)
                  n790 = local write "Report"(w1647) -> ()
                }
                frame "Acel_result" {
                  n791 = local read "Frecuencia de muestreo (Hz)"() -> (w1744:dbl)
                  n792 = local read "Pattern frequency (Hz)"() -> (w1743:dbl)
                  n793 = local read "Pattern amplitude (g)"() -> (w1742:dbl)
                  n794 = flat-sequence {
                    tunnel: w1745 -> [w1763]
                    tunnel: w1744 -> [w1761]
                    tunnel: w1743 -> [w1760]
                    tunnel: w1742 -> [w1759]
                    tunnel: [w1758] -> w1738
                    tunnel: [w1749] -> _
                    tunnel: [w1748] -> w1733
                    frame #0 {
                      n795 = for {
                        tunnel: w1763 -> [w1777] mode=indexing
                        tunnel: w1761 -> [w1773]
                        tunnel: w1760 -> [w1770]
                        tunnel: [w1771] -> w1768 mode=indexing
                        n796 = call-poly <vilib>:"Basic Averaged DC-RMS.vi"("signal in"=w1777) -> ("DC value"=w1778:dbl)  [unwired: 7 in, 3 out]
                        n797 = Subtract(x=w1777, y=w1778) -> (x-y=w1769:dbl[])
                        n798 = Divide(x=w1773, y=w1770) -> (x/y=w1774:dbl)
                        n799 = Array Size(array=w1769) -> (size(s)=w1775:i32)
                        n800 = Subtract(x=w1775, y=w1774) -> (x-y=w1776:dbl)
                        n801 = for {
                          N: w1776 -> [_]
                          tunnel: w1774 -> [w1780]
                          tunnel: [w1783] -> w1772 mode=indexing
                          tunnel: w1769 -> [w1782]
                          i -> [w1781]
                          n802 = Array Subset(array=w1782, index=w1781, length=w1780) -> (w1779:dbl[])
                          n803 = call-poly <vilib>:"RMS.vi"("X"=w1779) -> ("rms value"=w1783:dbl)  [unwired: 1 out]
                        }
                        n804 = call <vilib>:"Std Deviation and Variance.vi"("X"=w1772) -> ("mean"=w1771:dbl)  [unwired: 1 in, 2 out]
                      }
                      n805 = call <vilib>:"Std Deviation and Variance.vi"("X"=w1768) -> ("mean"=w1767:dbl)  [unwired: 1 in, 2 out]
                      n806 = Divide(x=w1759, y=w1767) -> (x/y=w1765:dbl)
                      n807 = Reciprocal(x=w1765) -> (1/x=w1762:dbl)
                      n808 = Multiply(x=w1762, y=1000.0) -> (x*y=w1755:dbl)
                      n809 = Number To Fractional String(number=w1755, precision (6)=i16 2) -> (F-format string=w1751:string)  [unwired: 2 in]
                      n810 = Divide(x=w1762, y=9.81) -> (x/y=w1758:dbl)
                      n811 = In Range and Coerce(upper limit=14.5, x=w1755, lower limit=7.5) -> (In Range?=w1749:bool)  [unwired: 1 out]
                      n812 = Select(t="\n\nACCELEROMETER CALIBRATED CORRECTLY\n------------------------------------------------------------------------ \n", s=w1749, f="\n\nCALIBRATION FAILED\nSENSITIVITY OUT OF RANGE (7,5-14,5)\n------------------------------------------------------------------------ \n") -> (s? t:f=w1750:string)
                      n813 = Concatenate Strings("\nAMPLITUDE CALIBRATION:\n\nSENSIVITY: ", w1751, w1750, "\r") -> (w1748:string)
                    }
                  }
                  n814 = local read "Report"() -> (w1741:string)
                  n815 = Concatenate Strings(w1733, w1741) -> (w1740:string)
                  n816 = local write "Report"(w1740) -> ()
                  "Calibration parameter" <- w1738
                }
              }
              n817 = Wait Until Next ms Multiple(millisecond multiple=u32 200 ("milliseconds to wait")) -> ()  [unwired: 1 out]
              n818 = Not(x=w1037) -> (.not. x?=w1043:bool)
              n819 = Concatenate Strings(w1039, w1041) -> (w1040:string)
              "Numeric" <- w1038
            }
            n820 = while {
              tunnel: [w1014] -> w994
              tunnel: w995 -> [w1014]
              i -> [w1011]
              stop <- w1012 stop-if-true
              n821 = Wait (ms)(milliseconds to wait=u32 1000) -> ()  [unwired: 1 out]
              n822 = Greater?(x=w1011, y=2) -> (0:w1012:bool)
            }
            n823 = local read "calibration log"() -> (w1001:path)
            n824 = Write to Text File(file (use dialog)=w1001, text=w994) -> ()  [unwired: 2 in, 3 out]
            n825 = flat-sequence {
              tunnel: w1000 -> [w1023]
              tunnel: w996 -> [w1022]
              tunnel: [w1023] -> w999
              tunnel: [w1022] -> w997
              frame #0 {
                # "Antes Accel. detected"
                n826 = local read "Accelerometer"() -> (w1020:i32)
                n827 = local read "Save calibration"() -> (w1019:bool)
                n828 = Add(x=w1020, y=7) -> (x+y=w1017:i32)
                n829 = Less Or Equal?(x=w1017, y=15) -> (x <= y?=w1018:bool)
                n830 = And(x=w1018, y=w1019) -> (x .and. y?=w1015:bool)
                n831 = case shown="True" w1015 {
                  tunnel: w1017 -> [_ w1024]
                  frame False {
                  }
                  frame True {
                    w1034 = "Parametros"  # Key 1
                    n832 = local read "configuration file path"() -> (w1026:path)
                    n833 = local read "Calibration parameter"() -> (w1025:dbl)
                    n834 = Number To Decimal String(number=w1024) -> (decimal integer string=w1035:string)  [unwired: 1 in]
                    n835 = Concatenate Strings(w1034, w1035) -> (w1028:string)
                    n836 = call <vilib>:"Open Config Data.vi"("create file if necessary (T)"=TRUE, "configuration file path"=w1026) -> ("error out"=w1029:errorcluster, "refnum"=w1030:T13)  [unwired: 1 in, 7 out]
                    n837 = call-poly <vilib>:"Write Key.vi"("section"="Adquisicion", "error in (no error)"=w1029, "value"=w1025, "key"=w1028, "refnum"=w1030) -> ("error out"=w1033:errorcluster, "refnum out"=w1032:T13)  [unwired: 3 in, 2 out]
                    n838 = call <vilib>:"Close Config Data.vi"("error in (no error)"=w1033, "refnum"=w1032) -> ()  [unwired: 8 in, 2 out]
                  }
                }
              }
            }
          }
          frame "UPS" {
            n839 = flat-sequence {
              tunnel: w1791 -> [w1803]
              tunnel: [w1803] -> w1790
              frame #0 {
                n840 = local read "Report"() -> (w1802:string)
                n841 = call "Reporting_datetime.vi"() -> ("String"=w1800:string)  [unwired: 11 in]
                n842 = Concatenate Strings(w1800, "\nSTATUS: UPS\n\n", w1802) -> (w1801:string)
                n843 = local write "Report"(w1801) -> ()
              }
            }
            n844 = node-c288() -> (w1798:T7)  [unwired: 4 in]
            n845 = timed-loop {
              timing: w1798 -> [_]
              timing-out: [_] -> w1797
              tunnel: w1796 -> [w1812]
              tunnel: w1790 -> [w1811]
              tunnel: [w1810] -> w1795
              tunnel: [w1809] -> w1794
              stop <- w1804 stop-if-true
              n846 = node-c288() -> ()  [unwired: 1 in, 1 out]
              n847 = xnode "Read/Write Control"("FPGA VI Reference In"=w1812, "error in"=w1811) -> ("FPGA VI Reference Out"=w1810:refnum<k20>, "error out"=w1809:errorcluster, "DC OK"=w1807:bool, "Chassis Temperature"=w1808:i16)
              n848 = call "ControlTemperatura.vi"("Chassis Temperature"=w1808) -> ("T fuera rango"=w1806:bool)  [unwired: 2 out]
              n849 = Not(x=w1806) -> (.not. x?=w1805:bool)
              n850 = And(x=w1807, y=w1805) -> (x .and. y?=w1804:bool)
              n851 = node-c288() -> ()  [unwired: 1 in, 1 out]
            }
            n852 = node-c288(w1797) -> ()  [unwired: 1 out]
          }
          frame "Diagnosis" {
            (unwired) "%Y/%m/%d %H:%M:%S" ("time format string (%c)")
            n853 = flat-sequence {
              tunnel: w1838 -> [w2049]
              tunnel: [w2049] -> w1837
              frame #0 {
                n854 = local read "Report"() -> (w2048:string)
                n855 = call "Reporting_datetime.vi"() -> ("String"=w2046:string)  [unwired: 11 in]
                n856 = Concatenate Strings(w2046, "\nSTATUS: AUTODIAGNOSIS\n\n", w2048) -> (w2047:string)
                n857 = local write "Report"(w2047) -> ()
              }
            }
            n858 = xnode "Invoke Method"("FPGA VI Reference In"=w1836, "error in"=w1837) -> ("FPGA VI Reference Out"=w1828:refnum<k20>, "error out"=w1829:errorcluster)  [unwired: 1 in]
            n859 = flat-sequence {
              tunnel: [w1862] -> w1835
              tunnel: [w1861] -> w1834
              tunnel: [w1852] -> w1833
              tunnel: [w1851] -> w1832
              tunnel: w1829 -> [w1840]
              tunnel: w1828 -> [w1841]
              tunnel: [w1844] -> w1824
              tunnel: [w1843] -> w1823
              tunnel: w1835 -> [w1886]
              tunnel: w1834 -> [w1887]
              tunnel: w1833 -> [w1884]
              tunnel: w1832 -> [w1883]
              tunnel: [w1885] -> w1831
              tunnel: [w1881] -> w1830
              tunnel: w1824 -> [w1876]
              tunnel: w1823 -> [w1875]
              tunnel: [w1872] -> w1822
              tunnel: w1831 -> [w1959]
              tunnel: w1830 -> [w1960]
              tunnel: w1822 -> [w1952]
              tunnel: [w1974] -> w1821
              tunnel: [w1973] -> w1820
              tunnel: [w2043] -> w1827
              tunnel: [w2044] -> w1818
              tunnel: w1821 -> [w2044]
              tunnel: w1820 -> [w2043]
              frame #0 {
                w1842 = sgl[] [] ("A1")
                n860 = local read "Frecuencia de muestreo y módulo CRIO"() -> (w1860:T3)
                n861 = local read "Escaneos de la FIFO por canal"() -> (w1857:u32)
                n862 = local read "Frecuencia de muestreo (Hz)"() -> (w1858:dbl)
                n863 = local read "Nº de acelerómetros"() -> (w1855:i32)
                n864 = Get Date/Time In Seconds() -> (seconds since 1Jan1904=→"Inicio diagnosis":timestamp)
                n865 = local read "Nº inductivos"() -> (w1856:i32)
                n866 = local read "Canal cero WS2"() -> (w1849:bool)
                n867 = local read "Canal cero WS1?"() -> (w1850:bool)
                n868 = local read "Count(mSec)"() -> (w1859:u32)
                n869 = xnode "Read/Write Control"("FPGA VI Reference In"=w1841, "error in"=w1840, "Fotocélula"=TRUE ("Adquirir")) -> ("FPGA VI Reference Out"=w1866:refnum<k20>, "error out"=w1865:errorcluster)
                n870 = Add(x=w1856, y=w1855) -> (x+y=w1854:i32)
                n871 = call "DMACalc.vi"("Number of Channels"=w1854, "Number of Samples"=w1857, "Rate (Hz)"=w1858) -> ("Block Size"=w1851:u32, "Time to Acquire Block (ms)"=w1852:i32, "Host Buffer Size"=w1853:u32)  [unwired: 6 in]
                n872 = xnode "Read/Write Control"("FPGA VI Reference In"=w1866, "error in"=w1865, "Data Rate"=w1860, "Digital?"=FALSE, "Count(mSec)"=w1859, "Canal cero WS1?"=w1850, "Canal cero WS2?"=w1849) -> ("FPGA VI Reference Out"=w1868:refnum<k20>, "error out"=w1867:errorcluster)
                n873 = xnode "Invoke Method"("FPGA VI Reference In"=w1868, "error in"=w1867, "Requested Depth"=w1853) -> ("FPGA VI Reference Out"=w1870:refnum<k20>, "error out"=w1869:errorcluster)  [unwired: 1 out]
                n874 = Open/Create/Replace File(file path (use dialog)=path "c:/diagnosis.bin" ("file (use dialog)"), operation (0:open)=T5."replace or create", access (0:read/write)=enum16{"read/write", "read-only", "write-only"}."read/write", disable buffering (F)=TRUE) -> (refnum out=w1844:refnum<file>, error out=w1843:errorcluster)  [unwired: 1 in, 2 out]
                n875 = xnode "Invoke Method"("FPGA VI Reference In"=w1870, "error in"=w1869) -> ("FPGA VI Reference Out"=w1862:refnum<k20>, "error out"=w1861:errorcluster)
                n876 = local write "A1"(w1842) -> ()
                n877 = local write "A2"(w1842) -> ()
                n878 = local write "A3"(w1842) -> ()
                n879 = local write "A4"(w1842) -> ()
                n880 = local write "A5"(w1842) -> ()
                n881 = local write "A6"(w1842) -> ()
                n882 = local write "A7"(w1842) -> ()
                n883 = local write "A8"(w1842) -> ()
                n884 = local write "I1"(w1842) -> ()
                n885 = local write "I2"(w1842) -> ()
              }
              frame #1 {
                n886 = while "Data Acquisition" {
                  tunnel: w1886 -> [w1915]
                  shift-right: [w1919] -> _
                  shift-left: u32 0 ("t") -> [w1894]
                  tunnel: w1884 -> [w1920]
                  tunnel: w1883 -> [w1918]
                  shift-right: [w1921] -> w1881
                  shift-left: w1887 -> [w1914]
                  tunnel: [w1916] -> w1885
                  tunnel: w1876 -> [w1892]
                  shift-right: [w1889] -> w1874
                  shift-left: w1875 -> [w1891]
                  tunnel: [w1890] -> w1873
                  stop <- w1917 stop-if-true
                  # "Detector de presencia"
                  # "Mide el tiempo de paso del tren y con ello se puede calcular\nla velocidad la unidad"
                  n887 = xnode "Invoke Method"("FPGA VI Reference In"=w1915, "error in"=w1914, "Number of Elements"=w1894, "Timeout (ms)"=0) -> ("FPGA VI Reference Out"=w1907:refnum<k20>, "error out"=w1906:errorcluster, "Data"=w1913:fxp<+/-,24,4>[], "Elements Remaining"=w1895:u32)
                  n888 = case "Data Ready" shown="Default" w1894 {
                    tunnel: w1920 -> [w1926 _]
                    tunnel: [w1924 u32 0 ("t")] -> w1919
                    tunnel: w1918 -> [w1927 _]
                    tunnel: w1895 -> [w1925 _]
                    tunnel: w1913 -> [_ w1941]
                    tunnel: w1891 -> [w1923 w1938]
                    tunnel: [w1923 w1936] -> w1889
                    tunnel: w1892 -> [w1922 w1935]
                    tunnel: [w1922 w1934] -> w1890
                    frame 0 {
                      n889 = Greater Or Equal?(x=w1925, y=w1927) -> (x >= y?=w1928:bool)
                      n890 = case shown="False" w1928 {
                        tunnel: [u32 0 ("Block Size") w1932] -> w1924
                        tunnel: [w1931 0 ("t")] -> w1929
                        tunnel: w1926 -> [w1931 _]
                        tunnel: w1927 -> [_ w1932]
                        frame False {
                        }
                        frame True {
                        }
                      }
                      n891 = call "WaitMinTimeBetweenCall.vi"("Minimum ms between calls"=w1929) -> ()  [unwired: 2 in]
                    }
                    frame Default {
                      n892 = To Single Precision Float(number=w1941) -> (single precision float=w1937:sgl[])
                      n893 = Write to Binary File(file (use dialog)=w1935, data=w1937, error in=w1938, 5:FALSE ("prepend array or string size? (T)"), 9:T6."little-endian" ("byte order (0:big-endian, network order)")) -> (refnum out=w1934:refnum<file>, error out=w1936:errorcluster)  [unwired: 2 out]
                    }
                  }
                  n894 = xnode ("CheckLate")("FPGA VI Reference In"=w1907, "error in"=w1906) -> ("FPGA VI Reference Out"=w1902:refnum<k20>, "error out"=w1911:errorcluster, "Buffer Underflow"=w1897:bool, "Buffer Overflow"=w1898:bool)
                  n895 = local read "Inicio diagnosis"() -> (w1899:timestamp)
                  n896 = Get Date/Time In Seconds() -> (seconds since 1Jan1904=w1900:timestamp)
                  n897 = To Double Precision Float(number=w1899) -> (double precision float=w1905:dbl)
                  n898 = To Double Precision Float(number=w1900) -> (double precision float=w1904:dbl)
                  n899 = local write "Buffer Overflow"(w1898) -> ()
                  n900 = Subtract(x=w1904, y=w1905) -> (x-y=w1908:dbl)
                  n901 = local write "Buffer Underflow"(w1897) -> ()
                  n902 = Greater?(x=w1908, y=1.0 ("Tiempo de adquisición")) -> (0:w1903:bool)
                  n903 = call "ErrorOverFlow.vi"("Buffer Overflow"=w1898) -> ("error out"=w1909:errorcluster)
                  n904 = call "ErrorUnderFlow.vi"("Buffer Overflow"=w1897) -> ("error out"=w1910:errorcluster)
                  n905 = Unbundle By Name(w1889) -> ("status"=w1888:bool)
                  n906 = Merge Errors(w1911, w1910, w1909) -> (w1893:errorcluster)
                  n907 = Unbundle By Name(w1893) -> ("status"=w1912:bool)
                  n908 = Compound Arithmetic op=OR(w1912, w1903, w1888) -> (w1917:bool)
                  n909 = case "Flush" shown="True" w1917 {
                    tunnel: w1902 -> [w1943 w1948]
                    tunnel: w1893 -> [w1944 w1947]
                    tunnel: [w1944 w1946] -> w1921
                    tunnel: [w1943 w1945] -> w1916
                    frame False {
                    }
                    frame True {
                      n910 = xnode "Invoke Method"("FPGA VI Reference In"=w1948, "error in"=w1947) -> ("FPGA VI Reference Out"=w1945:refnum<k20>, "error out"=w1946:errorcluster)
                    }
                  }
                }
                n911 = local read "Report"() -> (w1880:string)
                n912 = call "Reporting_error.vi"("error out 2"=w1881, "Concept"="FPGA ") -> ("Reporting"=w1882:string)  [unwired: 1 in]
                n913 = Close File(refnum=w1873, error in=w1874) -> (path=w1872:path)  [unwired: 1 out]
                n914 = Concatenate Strings(w1882, w1880) -> (w1877:string)
                n915 = local write "Report"(w1877) -> ()
              }
              frame #2 {
                n916 = xnode "Read/Write Control"("FPGA VI Reference In"=w1959, "error in"=w1960) -> ("FPGA VI Reference Out"=w1957:refnum<k20>, "error out"=w1958:errorcluster, "Direccion 0?"=w1956:bool)
                n917 = Read from Binary File(5:sgl 1.25, 9:T6."little-endian" ("byte order (0:big-endian, network order)"), 10:-1 ("count (1)"), 11:w1952) -> (0:w1950:errorcluster, 2:w1951:sgl[], 3:w1949:refnum<file>)  [unwired: 1 in, 2 out]
                "Diagnostic data" <- w1951
                n918 = local write "Direccion 0?"(w1956) -> ()
                n919 = Close File(refnum=w1949, error in=w1950) -> ()  [unwired: 2 out]
                n920 = Decimate 1D Array(w1951) -> (w1965:sgl[], w1962:sgl[], w1963:sgl[], w1964:sgl[], w1966:sgl[], w1967:sgl[], w1968:sgl[], w1969:sgl[], w1970:sgl[], w1971:sgl[])
                n921 = Build Array(w1965, w1962, w1963, w1964, w1966, w1967, w1968, w1969, w1970, w1971) -> (w1961:sgl[][])
                n922 = xnode "Read/Write Control"("FPGA VI Reference In"=w1957, "error in"=w1958, "Stop"=TRUE) -> ("FPGA VI Reference Out"=w1975:refnum<k20>, "error out"=w1976:errorcluster)
                n923 = for {
                  tunnel: w1961 -> [w1977] mode=indexing
                  i -> [w1978]
                  n924 = case shown="9" w1978 {
                    tunnel: w1977 -> [w1979 w1980 w1981 w1982 w1983 w1984 w1985 w1986 w1987 w1988 _]
                    frame 0 {
                      "A1" <- w1979
                    }
                    frame 1 {
                      "A2" <- w1980
                    }
                    frame 2 {
                      "A3" <- w1981
                    }
                    frame 3 {
                      "A4" <- w1982
                    }
                    frame 4 {
                      "A5" <- w1983
                    }
                    frame 5 {
                      "A6" <- w1984
                    }
                    frame 6 {
                      "A7" <- w1985
                    }
                    frame 7 {
                      "A8" <- w1986
                    }
                    frame 8 {
                      "I1" <- w1987
                    }
                    frame 9 {
                      "I2" <- w1988
                    }
                    frame 10, Default {
                    }
                  }
                }
                n925 = xnode "Invoke Method"("FPGA VI Reference In"=w1975, "error in"=w1976) -> ("FPGA VI Reference Out"=w1974:refnum<k20>, "error out"=w1973:errorcluster)
              }
              frame #3 {
                n926 = local read "error_RFID"() -> (w1990:errorcluster)
                n927 = local read "Puerto RFID"() -> (w2038:u16)
                n928 = local read "configuration file path"() -> (w2031:path)
                n929 = local read "IP RFID"() -> (w2039:string)
                n930 = local read "RFID_status"() -> (w2041:path)
                n931 = Unbundle By Name(w1990) -> ("status"=w1989:bool)
                n932 = call "Read_diagnosis_data.vi"("configuration file path"=w2031) -> ("acelerometros"=w2022:dbl, "WD"=w2035:dbl)  [unwired: 9 in]
                n933 = call "conexion_internet.vi"() -> ("Internet status"=w2005:string, "Internet connection"=→"Internet connection":bool)  [unwired: 10 in]
                n934 = call "RFID_connection.vi"("Estado_de_conexion"=w1989, "Puerto RFID"=w2038, "IP RFID"=w2039) -> ("RFID_connection_text"=w2004:string, "RFID connection"=→"RFID connection":bool)  [unwired: 7 in]
                n935 = call "show_tag_status.vi"("file path (dialog if empty)"=w2041) -> ("Output"=→"Last Train passes - RFIDs":T1, "train_passes_text"=w2003:string)  [unwired: 9 in]
                n936 = local read "Direccion 0?"() -> (w2034:bool)
                n937 = local read "I1"() -> (w2033:sgl[])
                n938 = local read "I2"() -> (w2032:sgl[])
                n939 = local read "A1"() -> (w2021:sgl[])
                n940 = local read "A2"() -> (w2020:sgl[])
                n941 = local read "A3"() -> (w2014:sgl[])
                n942 = local read "A4"() -> (w2015:sgl[])
                n943 = local read "A5"() -> (w2016:sgl[])
                n944 = local read "A6"() -> (w2017:sgl[])
                n945 = local read "A7"() -> (w2018:sgl[])
                n946 = local read "A8"() -> (w2019:sgl[])
                n947 = call "Wheel_detector_status.vi"("WD_offset"=w2035, "I2"=w2032, "I1"=w2033, "Direccion 0?"=w2034) -> ("WD_status"=w2002:string, "I2"=→"Wheel detector 2":bool, "I1"=→"Wheel Detector 1":bool)  [unwired: 5 in]
                n948 = call "Accelerometer_status.vi"("Number"=1, "Acc_offset"=w2022, "Accelerometer"=w2021) -> ("Accelerometer_status"=w2001:string, "Accelerometer"=→"Accelerometer 1":bool)  [unwired: 7 in]
                n949 = call "Accelerometer_status.vi"("Number"=2, "Acc_offset"=w2022, "Accelerometer"=w2020) -> ("Accelerometer_status"=w2000:string, "Accelerometer"=→"Accelerometer 2":bool)  [unwired: 7 in]
                n950 = call "Accelerometer_status.vi"("Number"=3, "Acc_offset"=w2022, "Accelerometer"=w2014) -> ("Accelerometer_status"=w1999:string, "Accelerometer"=→"Accelerometer 3":bool)  [unwired: 7 in]
                n951 = call "Accelerometer_status.vi"("Number"=4, "Acc_offset"=w2022, "Accelerometer"=w2015) -> ("Accelerometer_status"=w1998:string, "Accelerometer"=→"Accelerometer 4":bool)  [unwired: 7 in]
                n952 = call "Accelerometer_status.vi"("Number"=5, "Acc_offset"=w2022, "Accelerometer"=w2016) -> ("Accelerometer_status"=w1997:string, "Accelerometer"=→"Accelerometer 5":bool)  [unwired: 7 in]
                n953 = call "Accelerometer_status.vi"("Number"=6, "Acc_offset"=w2022, "Accelerometer"=w2017) -> ("Accelerometer_status"=w1996:string, "Accelerometer"=→"Accelerometer 6":bool)  [unwired: 7 in]
                n954 = call "Accelerometer_status.vi"("Number"=7, "Acc_offset"=w2022, "Accelerometer"=w2018) -> ("Accelerometer_status"=w1995:string, "Accelerometer"=→"Accelerometer 7":bool)  [unwired: 7 in]
                n955 = call "Accelerometer_status.vi"("Number"=8, "Acc_offset"=w2022, "Accelerometer"=w2019) -> ("Accelerometer_status"=w1994:string, "Accelerometer"=→"Accelerometer 8":bool)  [unwired: 7 in]
                n956 = local read "Report"() -> (w1993:string)
                n957 = Concatenate Strings(w2005, w2004, w2003, w2002, w2001, w2000, w1999, w1998, w1997, w1996, w1995, w1994, w1993) -> (w1992:string)
                n958 = property on="Report" class="Str"("Value"=w1992) -> ()  [unwired: 2 in, 2 out]
              }
            }
            n959 = local write "error_RFID"(errorcluster {"status"=FALSE, "code"=0, "source"=""} ("error_RFID")) -> ()
            n960 = Get Date/Time In Seconds() -> (seconds since 1Jan1904=w1826:timestamp)
            n961 = Format Date/Time String(seconds (now)=w1826) -> (date/time string=→"Last time checked":string)  [unwired: 2 in]
          }
        }
        "error manipulacion archivos" <- w111
        n962 = local read "Parar la aplicación"() -> (w109:bool)
      }
      n963 = local read "RFID NEM on?"() -> (w82:bool)
      n964 = case shown="True" w82 {
        frame False {
        }
        frame True {
          w90 = T14 {"IP"="169.254.1.1", "Port"=5084, "ReaderConfigFile"=path "", "ROspecConfigFile"=path ""}  # RFID Configuration
          w94 = path "" ("ReaderConfigFile")
          # "Loop RFID reader"
          n965 = local read "Puerto RFID"() -> (w92:u16)
          n966 = local read "IP RFID"() -> (w93:string)
          n967 = Bundle By Name(cluster=w90, "IP"=w93, "Port"=w92, "ReaderConfigFile"=w94, "ROspecConfigFile"=w94) -> (w91:T14)
          n968 = while {
            tunnel: w91 -> [w96]
            stop <- w97 stop-if-true
            n969 = local read "Parar la aplicación"() -> (w97:bool)
            n970 = call "IF2_Reader.vi"("Stop"=w97, "RFID Configuration"=w96) -> ("error out"=w98:errorcluster, "connection ID"=→"connection ID":refnum<k5>)  [unwired: 8 in]
            n971 = case shown="Error" w98 {
              tunnel: w98 -> [_ w100]
              tunnel: [TRUE ("RFIDStatus") FALSE ("RFIDStatus")] -> _
              frame No Error {
              }
              frame Error {
                n972 = call "Reporting_error.vi"("error out 2"=w100, "Concept"="Passive RFID") -> ("Reporting"=w102:string)  [unwired: 1 in]
                n973 = local read "Report"() -> (w103:string)
                n974 = Concatenate Strings(w102, w103) -> (w101:string)
                n975 = local write "Report"(w101) -> ()
                "error_RFID" <- w100
              }
            }
          }
        }
      }
      n976 = xnode "Close FPGA VI Reference"("FPGA VI Reference In"=w85, "error in"=w84) -> ("error out"=→"error FPGA":errorcluster)
    }
    frame #3 {
      n977 = call "LH6HD.vi"("Action"=enum16{"Init", "Start", "Read", "Stop", "Exit"}."Stop") -> ("error out"=→"RFID_LR6_Error":errorcluster)  [unwired: 9 in, 1 out]
    }
  }
